vi "Text control 2 v6.4.vi"() -> ()   [LabVIEW 2016]
panel:
  in  "Tab Control":enum32{"Main", "Other parameters"}(tab)
  out "Line running":i32
  out "Total lines":i32
  out "Path":path=path "C:/users/rlp38/09Apr2009LTtesting/test2.txt"
  out "I vs Vg":cluster{"Y data in":dbl[], "X data in":dbl[]}[](graph)
  out "Is max":dbl format="%.2e"
  out "Id max":dbl format="%.2e"
  out "Ig max":dbl format="%.2e"
  out "Imax vs time":cluster{"Y data in":dbl[], "X data in":dbl[]}[](graph)
  out "Imin vs time":cluster{"Y data in":dbl[], "X data in":dbl[]}[](graph)
  out "I vs Vd":cluster{"Y data in":dbl[], "X data in":dbl[]}[](graph)
  in  "Script":string="#pulsedstressV d 0.03 20 0 0.5 0.0827 5\n#\n#itime m\n#gaterangemode a\n#drainrangemode a\n#pulsed on 0.05 0 0.02\n#transfer d -10 40 1 5 40 35\n#transfer d -10 40 1 5 40 35\n#transfer d -10 40 1 5 40 35\n#output d 0 40 20 0 40 1\n#\n#\n#sample 1 0.008 221 6 0.003\n#samplei 400e-6 200 6 0.002 0.1\n#vsu2pulse -10 4\n#\n#stressV 0.016 0.03 2e-4 0.1e-3 11\n#stressI 220e-7 0.08 15\n#transfer s -1 1 0.5 -0.005 0.005 0.005\n#output s 0 0 0 -0.008 0.008 0.002"
  out "Command running:":string
  out "Serial port data":string
  out "Elapsed Time":dbl caption="Elapsed Time (s)"
  in  "Time Units":u16(ring)=1 items=["Seconds", "Minutes", "Hours"]
  in  "Time Offset":dbl caption="Set Start Time (s)"
  in  "Reset":bool
  in  "Auto Reset":bool
  in  "integration time":u32(slide) max=2 step=1 scale=0.0..2.0
  out "Is on":dbl format="%.2e"
  out "Id on":dbl format="%.2e"
  out "Ig on":dbl format="%.2e"
  out "Ion vs time":cluster{"Y data in":dbl[], "X data in":dbl[]}[](graph)
  out "Ioff vs time":cluster{"Y data in":dbl[], "X data in":dbl[]}[](graph)
  out "Ig min":dbl format="%.2e"
  out "Id min":dbl format="%.2e"
  out "Is min":dbl format="%.2e"
  out "Is off":dbl format="%.2e"
  out "Id off":dbl format="%.2e"
  out "Ig off":dbl format="%.2e"
  in  "Integration time (long)":dbl=0.32 min=0.04 max=2.0 step=0.02 format="%.2f"
  in  "Integration time (short)":dbl=0.0019 min=8e-05 max=0.0019 step=8e-05 format="%^.0e"
  in  "Drain: Compliance":dbl=0.001 format="%.8f"
  in  "Gate: Compliance":dbl=0.001 format="%.8f"
  in  "Interrupt scan":bool
  in  "Interrupt program":bool
  in  "Plot output curve extrema vs time":bool
  in  "Plot transfer curve extrema vs time":bool
  in  "Gate Range\nmode":u16(ring) items=["Auto", "Limited", "Fixed"]
  in  "Gate Range":u8(slide)=6 max=11 scale=0.0..11.0
  in  "Source/Drain\nRange mode":u16(ring) items=["Auto", "Limited", "Fixed"]
  in  "Source/Drain Range":u8(slide)=6 max=11 scale=0.0..11.0
  in  "Panel Controls":T1={"Emergency Stop"=refnum, "TransGraph Max"=1e-05, "Text/Graph (text=false)"=TRUE} {"TransGraph Max" format="%.2e"}
  in  "Panel Controls 2":T2={"Emergency Stop"=refnum, "TransGraph Max"=1e-05, "Text/Graph (text=false)"=TRUE, "TransGraph Min"=1e-11} {"TransGraph Min" format="%.2e"; "TransGraph Max" format="%.2e"}
  out "error out":errorcluster
  in  "Delay before read (ms)":u32=1000
  in  "byte count":u32=64
  in  "Serial End Mode for Reads":u16(ring)=2 items=["None", "LastBit", "TermChar"]
  in  "Timeout (ms)":u32=10000
  in  "Enable Termination\nChar (T)":bool=TRUE
  in  "Termination char\n(0xA = '\\n' = LF)\n(0xD = '\\r' = CR)":u8=13 format="%.0x"
  in  "flow control":u16(ring) items=["None"=0, "XON/XOFF"=1, "RTS/CTS"=2, "DTR/DSR"=4]
  in  "stop bits":u16(ring)=10 items=["1.0"=10, "1.5"=15, "2.0"=20]
  in  "parity":u16(ring) items=["None", "Odd", "Even", "Mark", "Space"]
  in  "data bits":u16=8 min=5 max=8 step=1
  in  "VISA resource name":refnum<visa-resource-name>="COM6"
  in  "baud rate":u32=9600
  out "Timings Indicator":T3
  in  "Timings (overwritten by the Front Panel)":T4={"integration time"=0, "Short/Long integration time"=0.00064, "hold time (sec)"=0.0, "delay time (sec)"=0.0, "Step Time (0 disables)"=0.0, "sweep method"=0, "Pulse period"=0.005, "Base voltage"=0.0, "Pulse width"=0.0005} {"Pulse width" min=0.0005 max=0.1 step=0.0001 format="%.4f"; "Base voltage" format="%^.4e"; "Pulse period" min=0.005 max=1.0 step=0.0001 format="%.4f"; "sweep method" items=["Continuous", "Pulsed"]; "Step Time (0 disables)" format="%.2f"; "delay time (sec)" format="%.4f"; "hold time (sec)" format="%.4f"; "Short/Long integration time" format="%^.0e"; "integration time" scale=0.0..2.0}
  in  "SMU4":cluster{"on/off":bool, "Voltage":dbl} {"Voltage" min=-100.0 max=100.0 format="%.2f"}
  in  "Full Reset":bool
  in  "Standby":T5
  in  "Gate":T6={"Gate Start"=0.0, "Gate Stop"=2.0, "Gate Step (linear only)"=1.0, "Gate Compliance"=0.0001, "Gate PComp"=0.0, "Range mode"=0, "Range"=6} {"Range" max=11 scale=0.0..11.0; "Range mode" items=["Auto", "Limited", "Fixed"]; "Gate PComp" format="%^.2e"; "Gate Compliance" format="%^.2e"; "Gate Step (linear only)" format="%^.4e"; "Gate Stop" format="%^.4e"; "Gate Start" format="%^.4e"}
  in  "Drain 2":T7={"Drain Start"=0.0, "Drain Stop"=2.0, "Drain Compliance"=0.0001, "Drain Step"=1.0, "Drain PComp"=0.0, "Range mode"=0, "Range"=6} {"Range" max=11 scale=0.0..11.0; "Range mode" items=["Auto", "Limited", "Fixed"]; "Drain PComp" format="%^.2e"; "Drain Step" format="%^.4e"; "Drain Compliance" format="%^.2e"; "Drain Stop" format="%^.4e"; "Drain Start" format="%^.4e"}
  # "Time"
  # "Syntax:\nitime [s|m|l] time(sec): [s|m|l] determines the integration time setting (small|medium|long) and time sets the value.\nNOTE: The value of the integration time has to be within the range allowed by its category (s|m|l), otherwise, the closest value will be used. (e.g. if the category is set to short but the time value is very long, the actual value used will be the maximum short integration time.\nIntegration times:\n    Short: Default: 640 us. Range: 8E-5 - 1.92E-3 seconds.\n    Medium: Fixed at 1 NPL cycle (0.02 seconds).\n    Long: Default: 16 NPL cycles (0.32 seconds). Range: 2-100 NPL cycles (0.04 seconds - 2 seconds).\ngaterangemode [a|l|f]\ndrainrangemode [a|l|f]\npulsed [on|off] PulsePeriod(sec) PulseBaseVoltage PulseONWidth(sec)\nstandby [on l off]\nwait NumMilliseconds\nwait-min NumMinutes\n# texthere = comment\ntransfer [s|d] VgStart VgStop VgStep VdStart VdStop VdStep\noutput [s|d] VgStart VgStop VgStep VdStart VdStop VdStep\nsample Vg Vd NumSamples Time(s) SampleInterval(s)\nsamplei Idg NumSamples Time(s) SampleInterval(s) VDGcompliance\n100 samples is approximately 13 seconds with medium integration\n# if in doubt use SampleInterval(s) = 0.004\nstressV VG VD IGcompliance IDcompliance Duration(sec)\nstressI IDG VDGcompliance Duration(sec)\nvsu2pulse Bias Duration(s)\npulsedstressV [s|d] VEstop VgON VgOFF Period(s) PulseONwidth(s) Vd\nsample-fpp Vg Vd NumSamples Time\nresample-fpp Vg Vd\ntransfer-fpp [s|d] VgStart VgStop VgStep VdStart VdStop VdStep\noutput-fpp [s|d] VgStart VgStop VgStep VdStart VdStop VdStep\nserial SerialPortCommand"
  # "1\n2\n3\n4\n5\n6\n7\n8\n9\n10\n11\n12\n13\n14\n15\n16\n17\n18\n19\n20"
  # "Serial port settings"
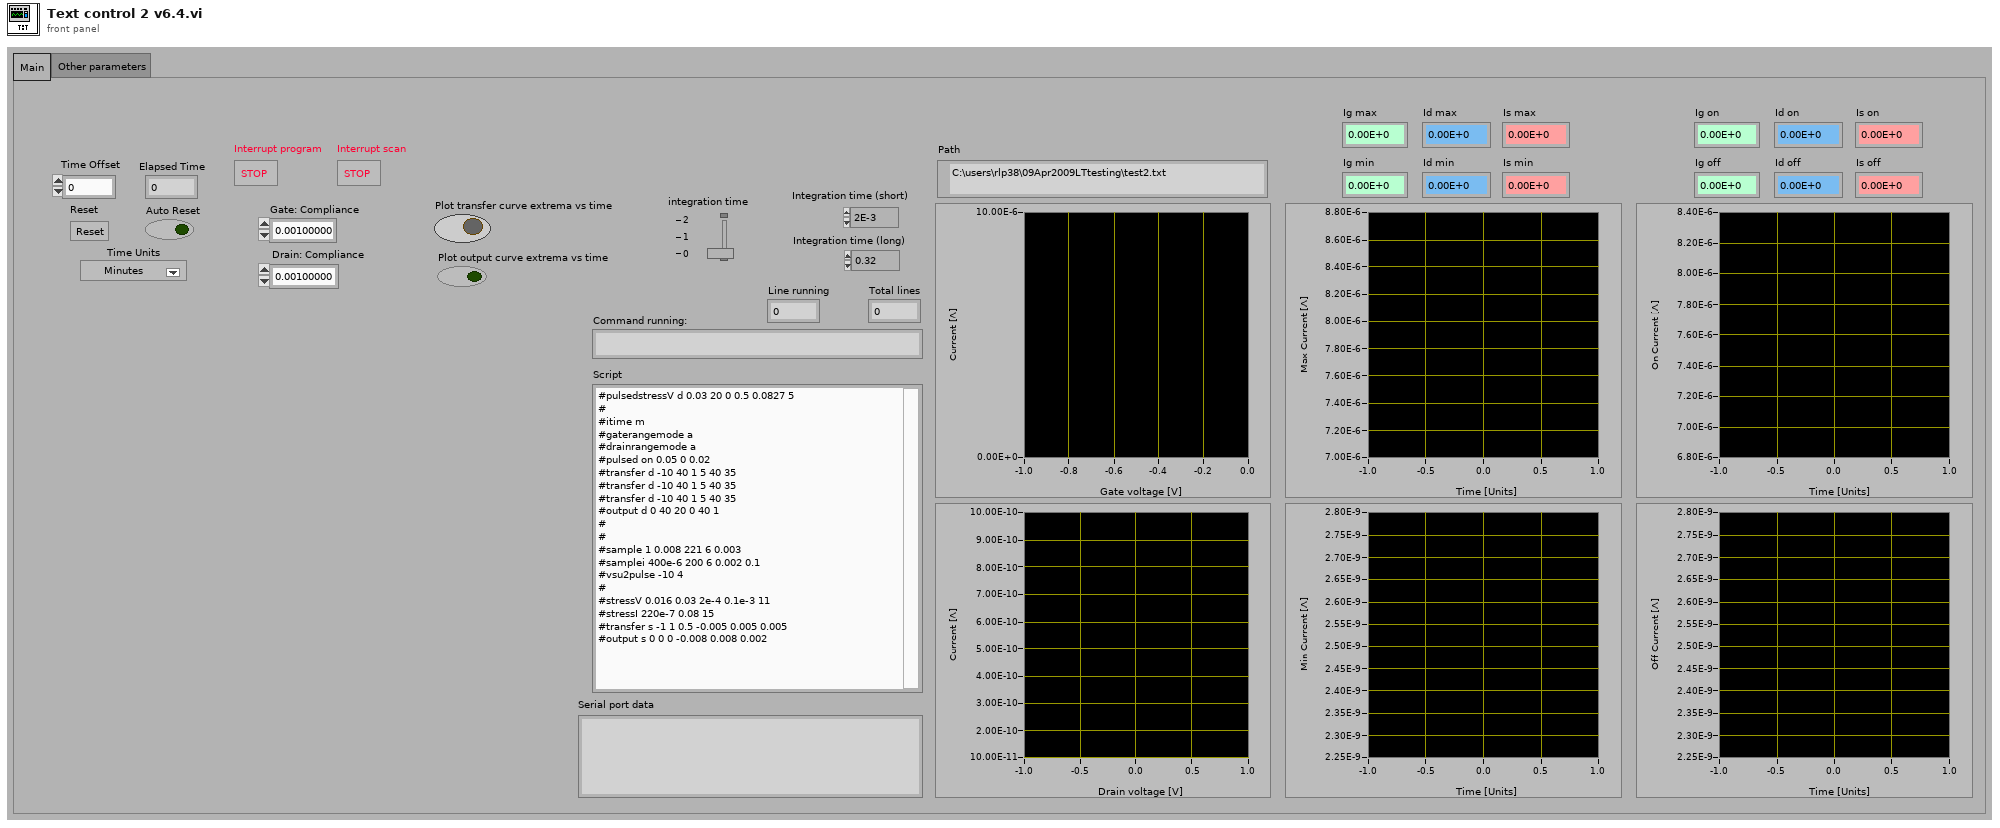
[diagram p1: front panel]
types:
  T1 = cluster{"Emergency Stop":refnum<vi>, "TransGraph Max":dbl, "Text/Graph (text=false)":bool}
  T2 = cluster{"Emergency Stop":refnum<vi>, "TransGraph Max":dbl, "Text/Graph (text=false)":bool, "TransGraph Min":dbl}
  T3 = cluster{"integration time (0:s, 1:m, 2:l)":u32, "Short/Long integration time":dbl, "hold time (sec)":dbl, "delay time (sec)":dbl, "Step Time (0 disables)":dbl, "sweep method":u16, "Pulse period":dbl, "Base voltage":dbl, "Pulse width":dbl}
  T4 = cluster{"integration time":u32, "Short/Long integration time":dbl, "hold time (sec)":dbl, "delay time (sec)":dbl, "Step Time (0 disables)":dbl, "sweep method":u16, "Pulse period":dbl, "Base voltage":dbl, "Pulse width":dbl}
  T5 = cluster{"Gate Standby":bool, "Drain Standby":bool}
  T6 = cluster{"Gate Start":dbl, "Gate Stop":dbl, "Gate Step (linear only)":dbl, "Gate Compliance":dbl, "Gate PComp":dbl, "Range mode":u16, "Range":u8}
  T7 = cluster{"Drain Start":dbl, "Drain Stop":dbl, "Drain Compliance":dbl, "Drain Step":dbl, "Drain PComp":dbl, "Range mode":u16, "Range":u8}
  T8 = enum16{"open", "replace", "create", "open or create", "replace or create", "replace or create with confirmation"}
  T9 = cluster{"V2 Start":dbl, "V2 Step":dbl, "Number of points":i32}
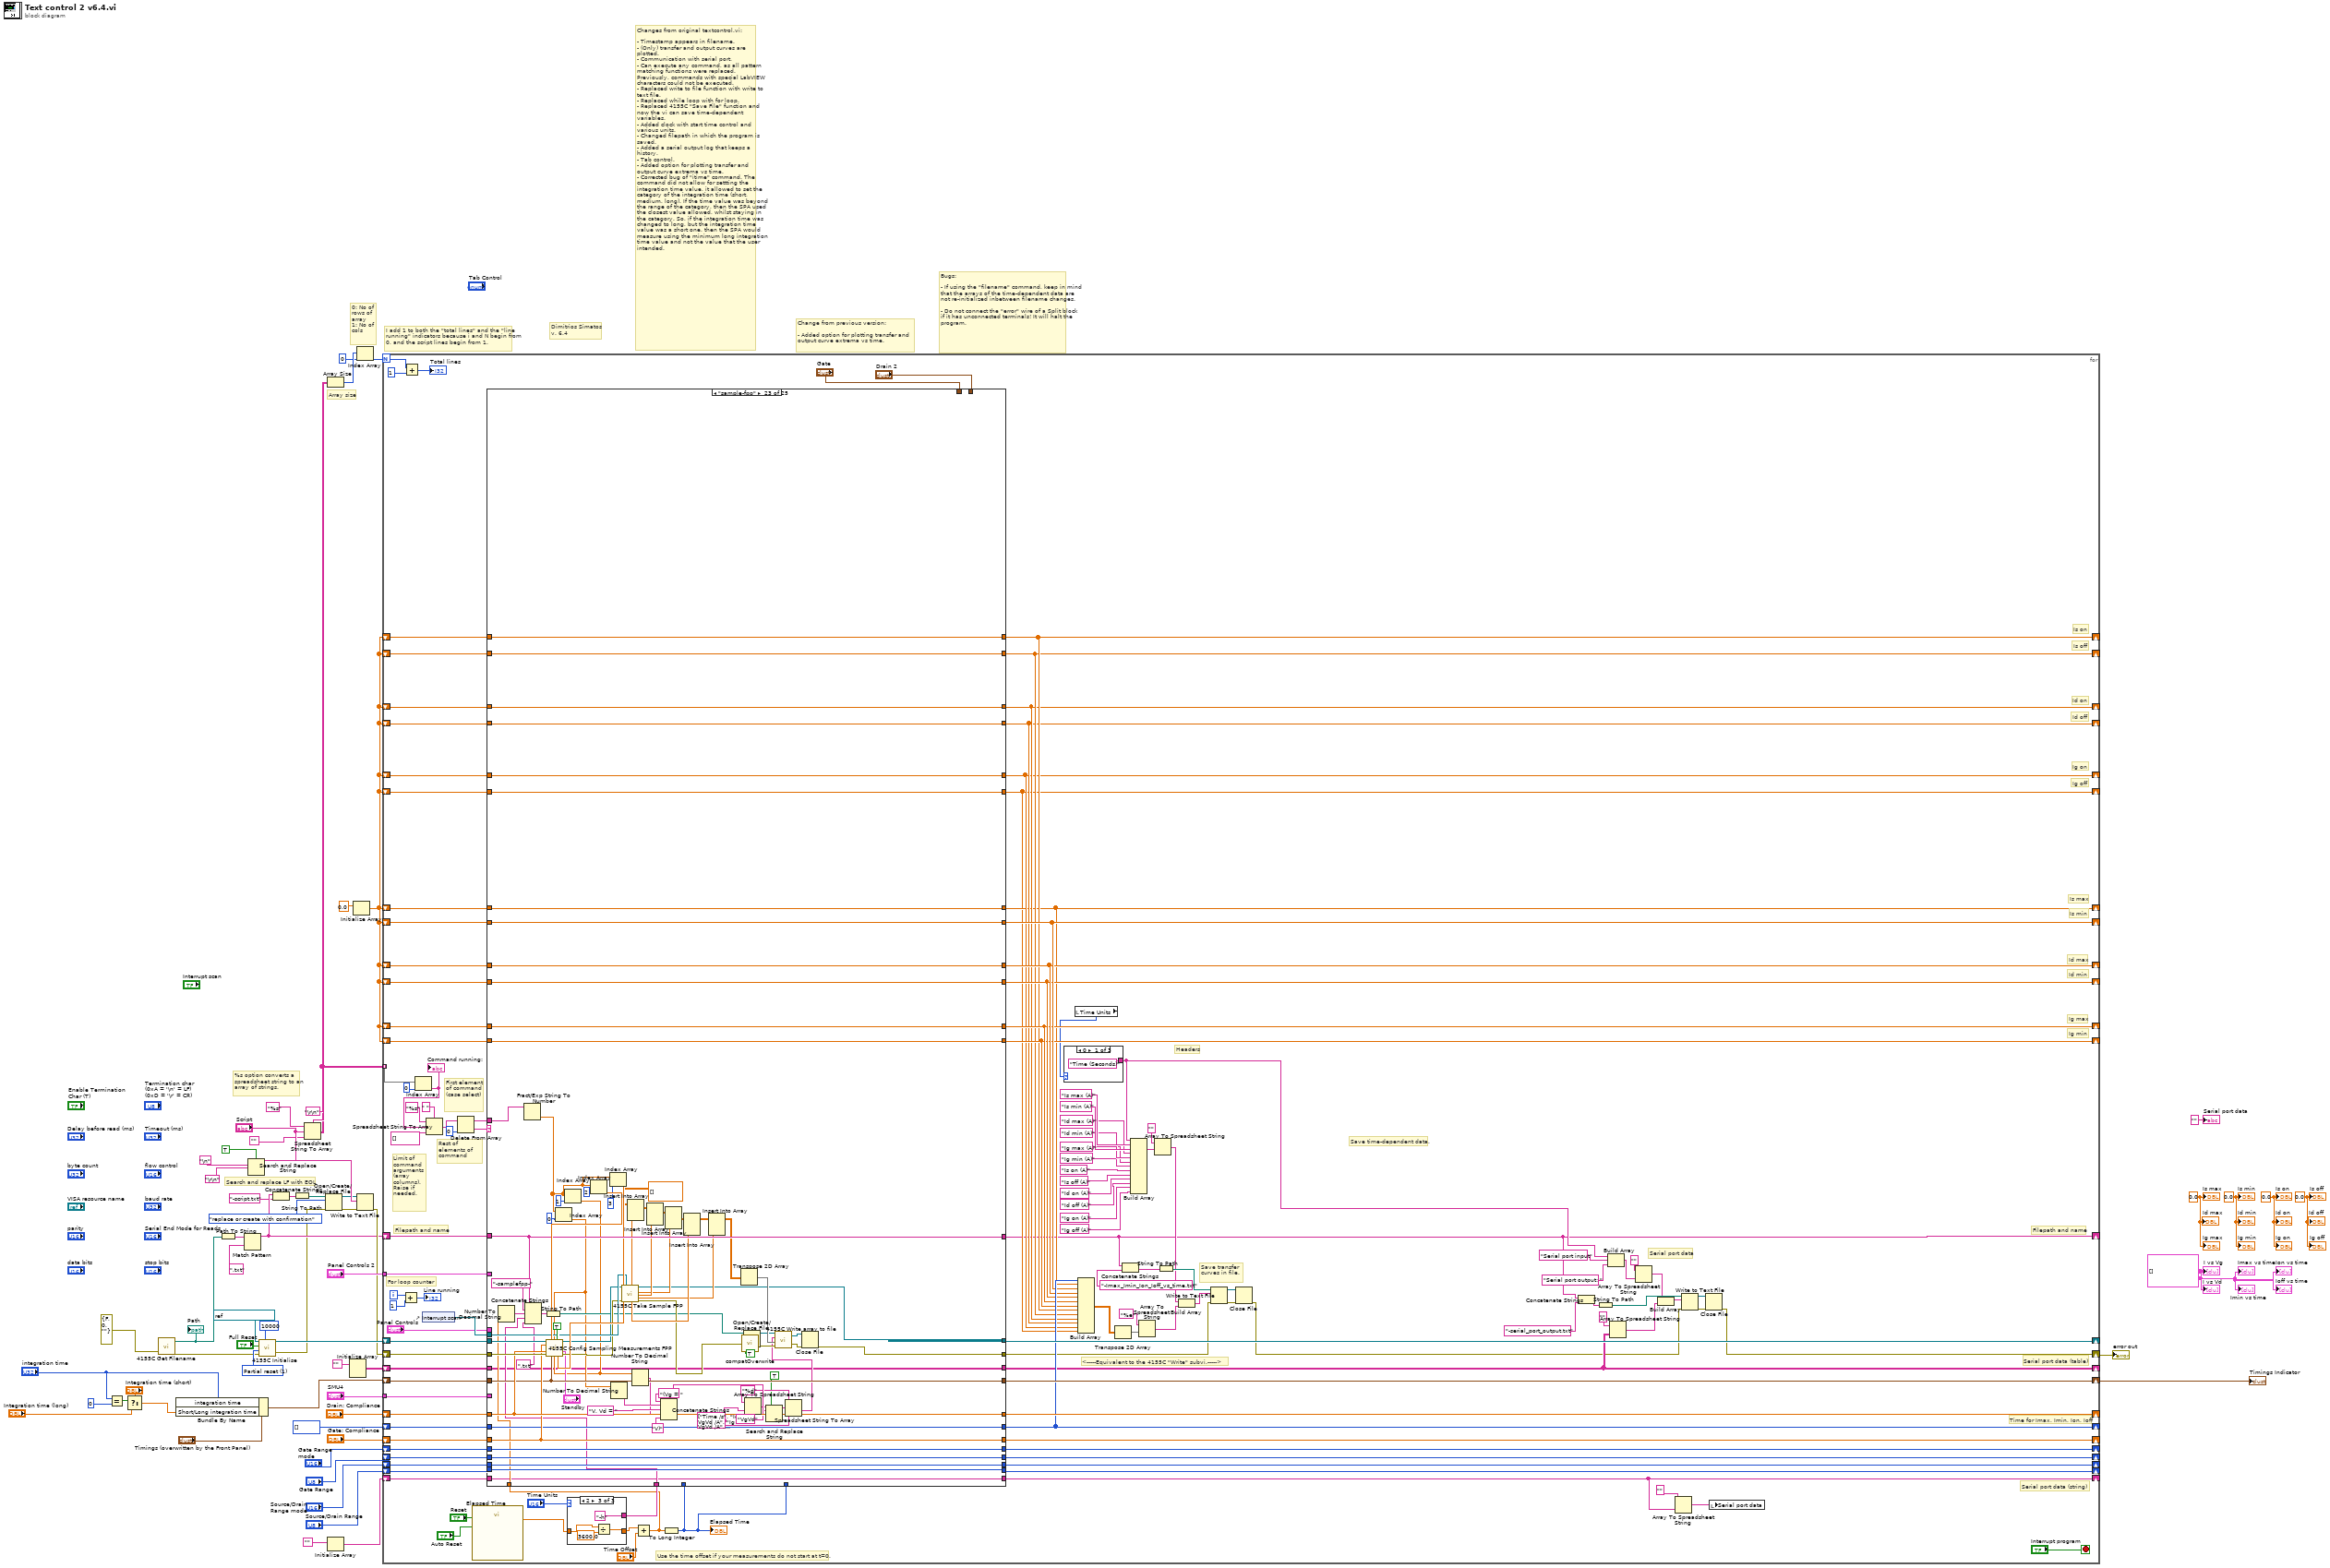
[diagram p0: block diagram]
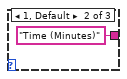
[diagram p2: hidden frame]
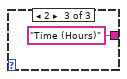
[diagram p3: hidden frame]
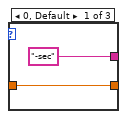
[diagram p4: hidden frame]
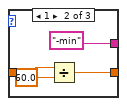
[diagram p5: hidden frame]
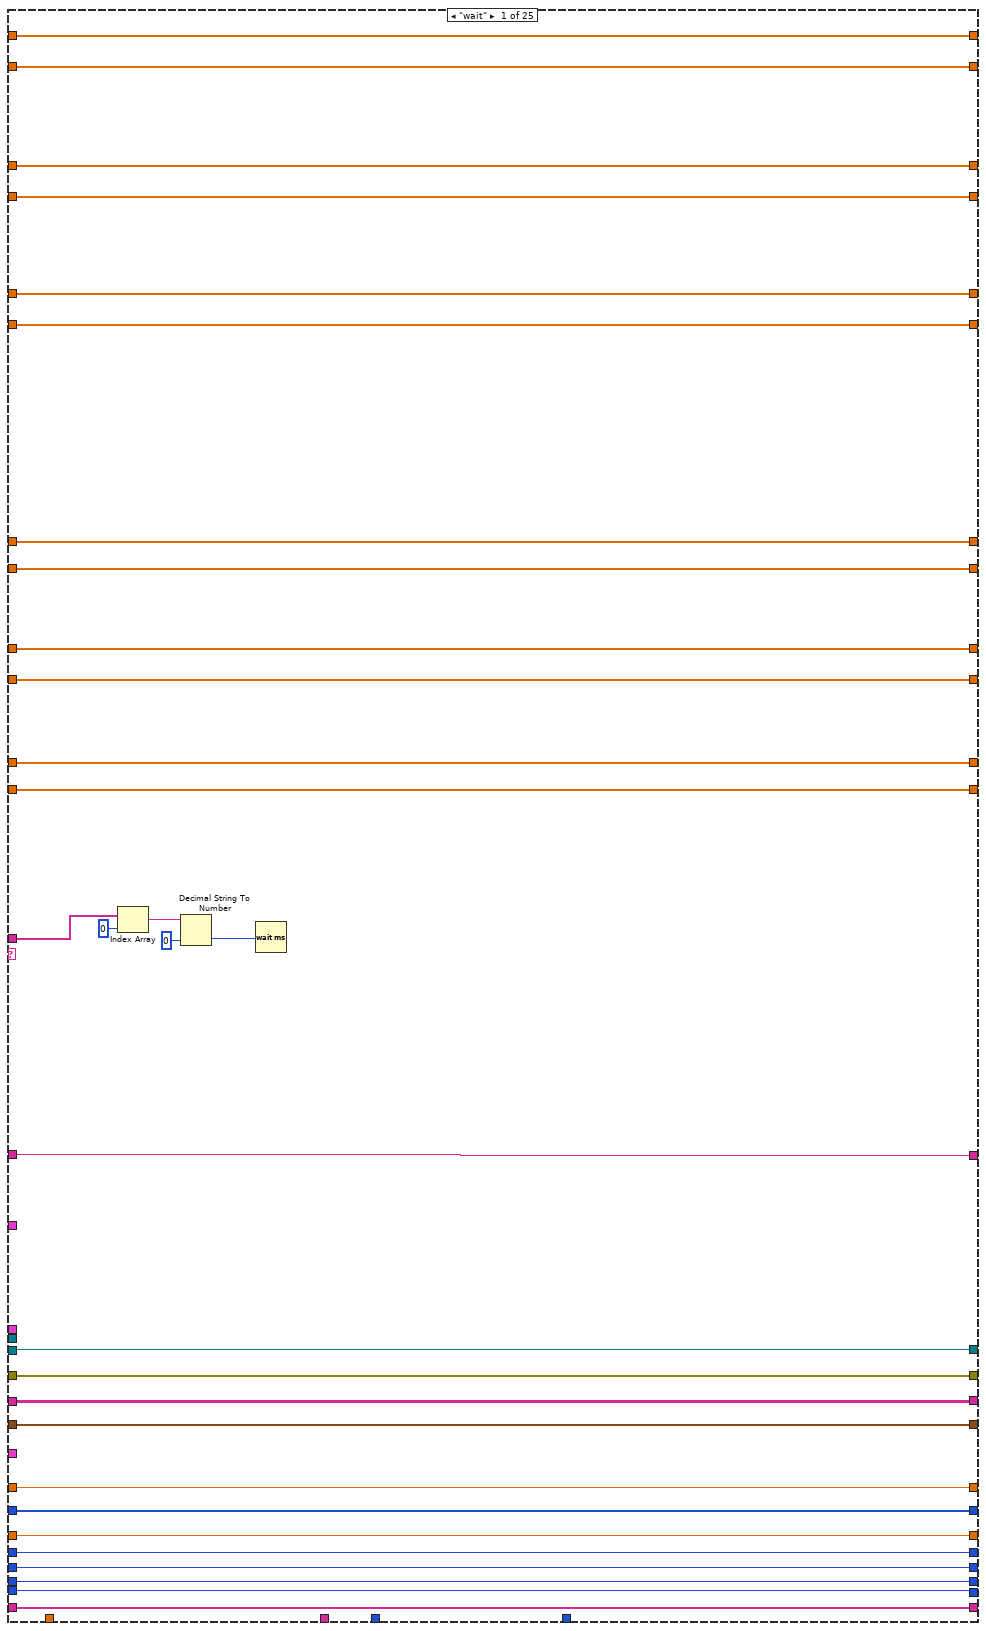
[diagram p6: hidden frame]
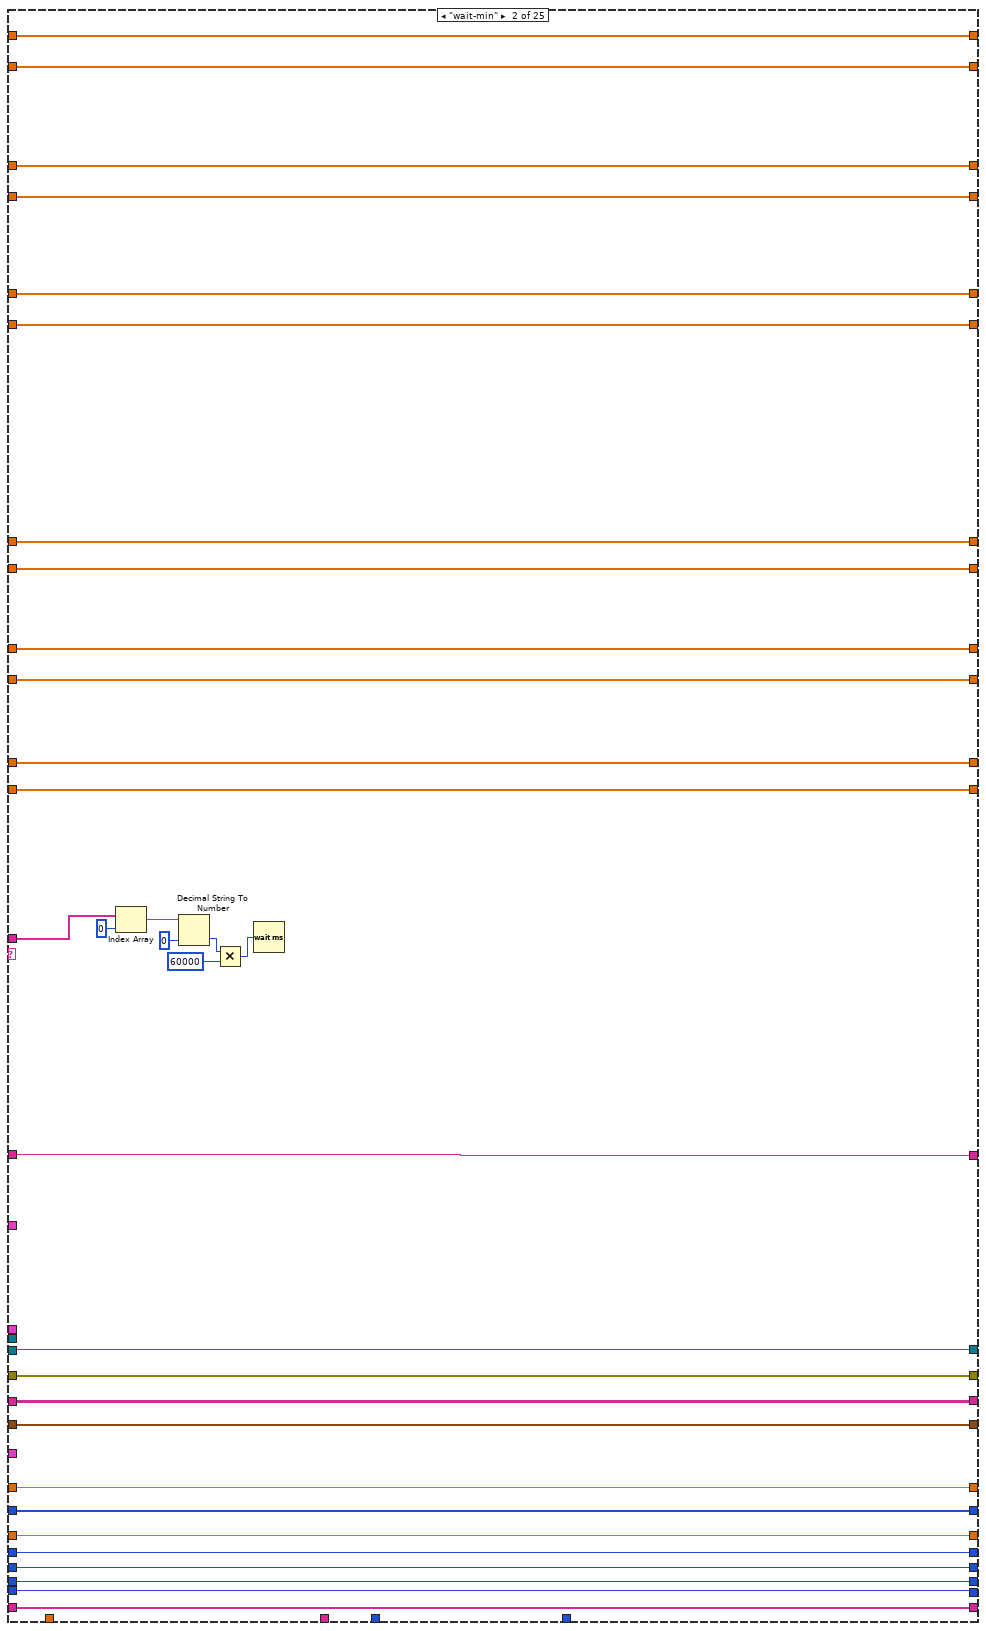
[diagram p7: hidden frame]
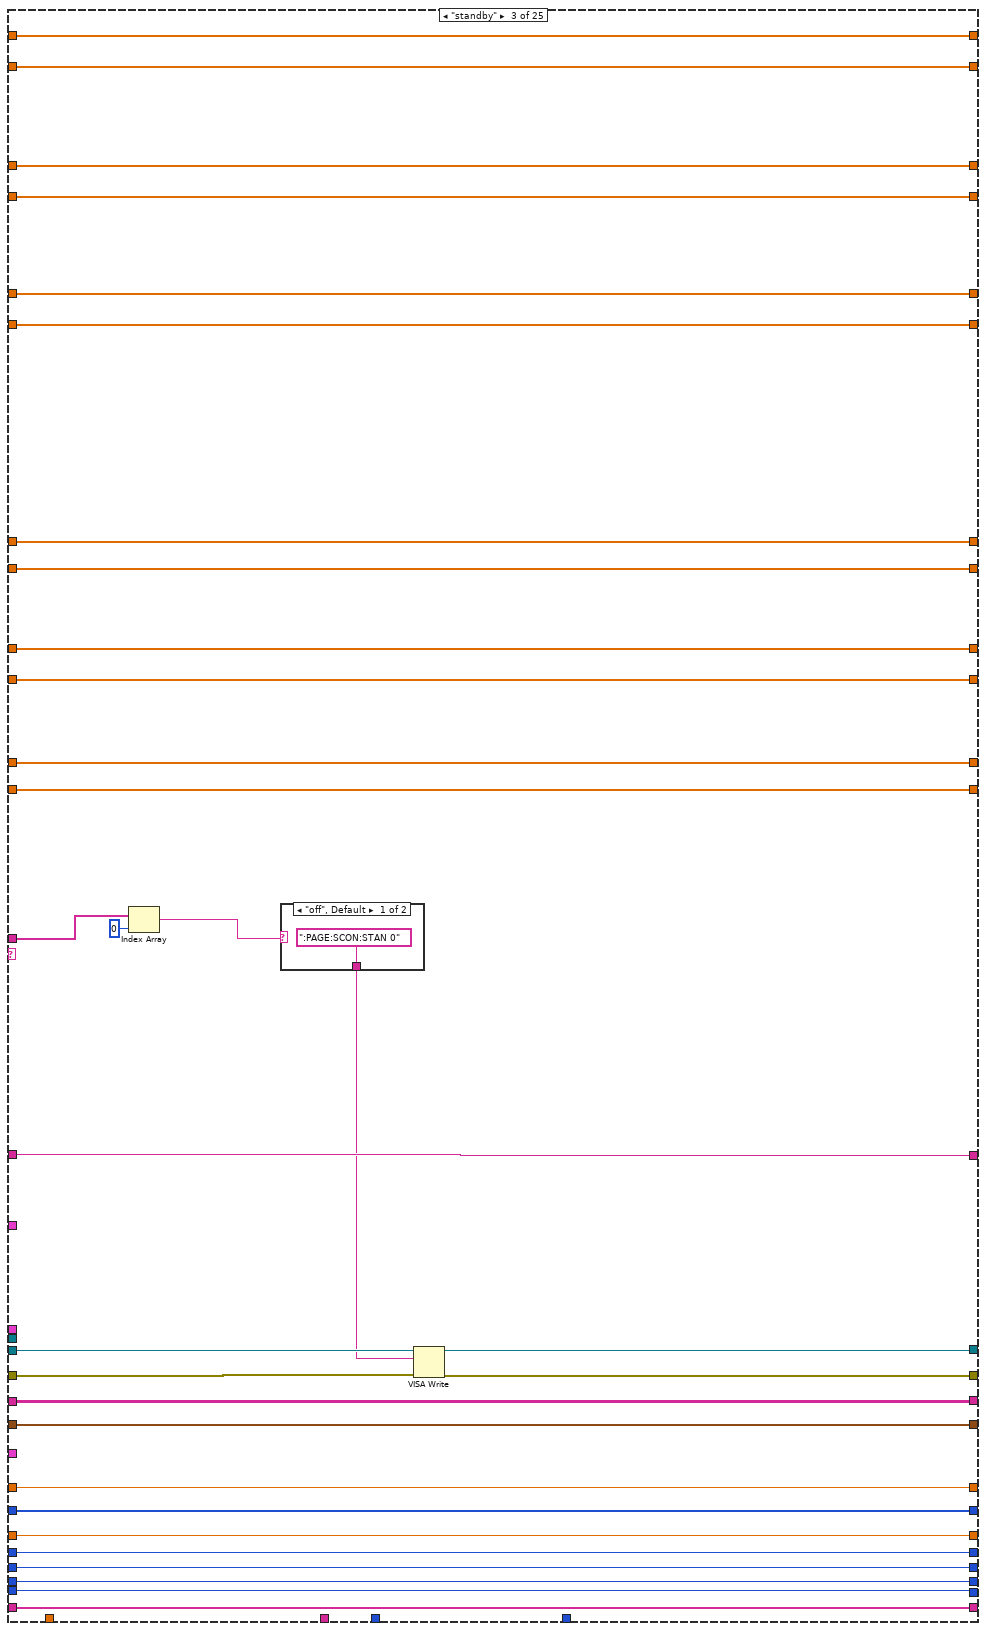
[diagram p8: hidden frame]
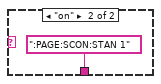
[diagram p9: hidden frame]
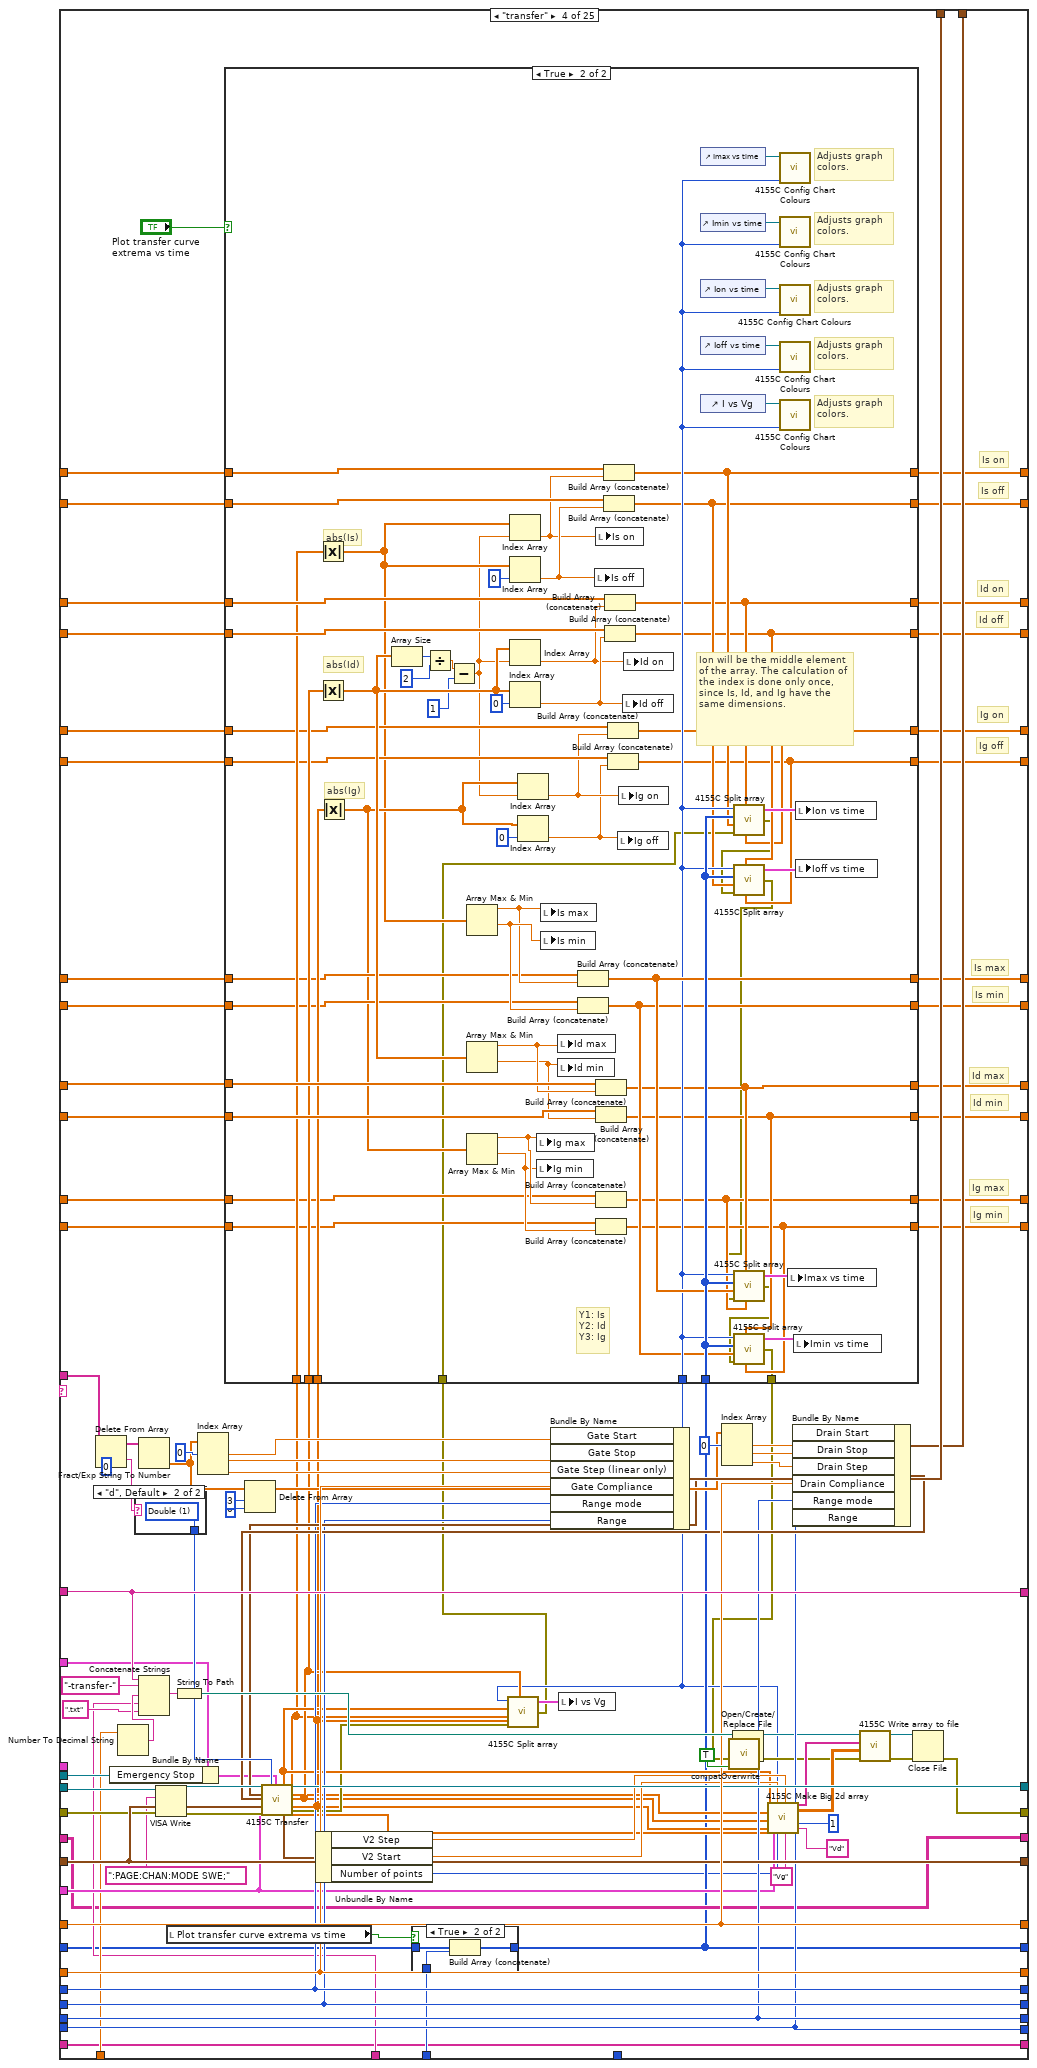
[diagram p10: hidden frame]
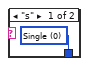
[diagram p13: hidden frame]
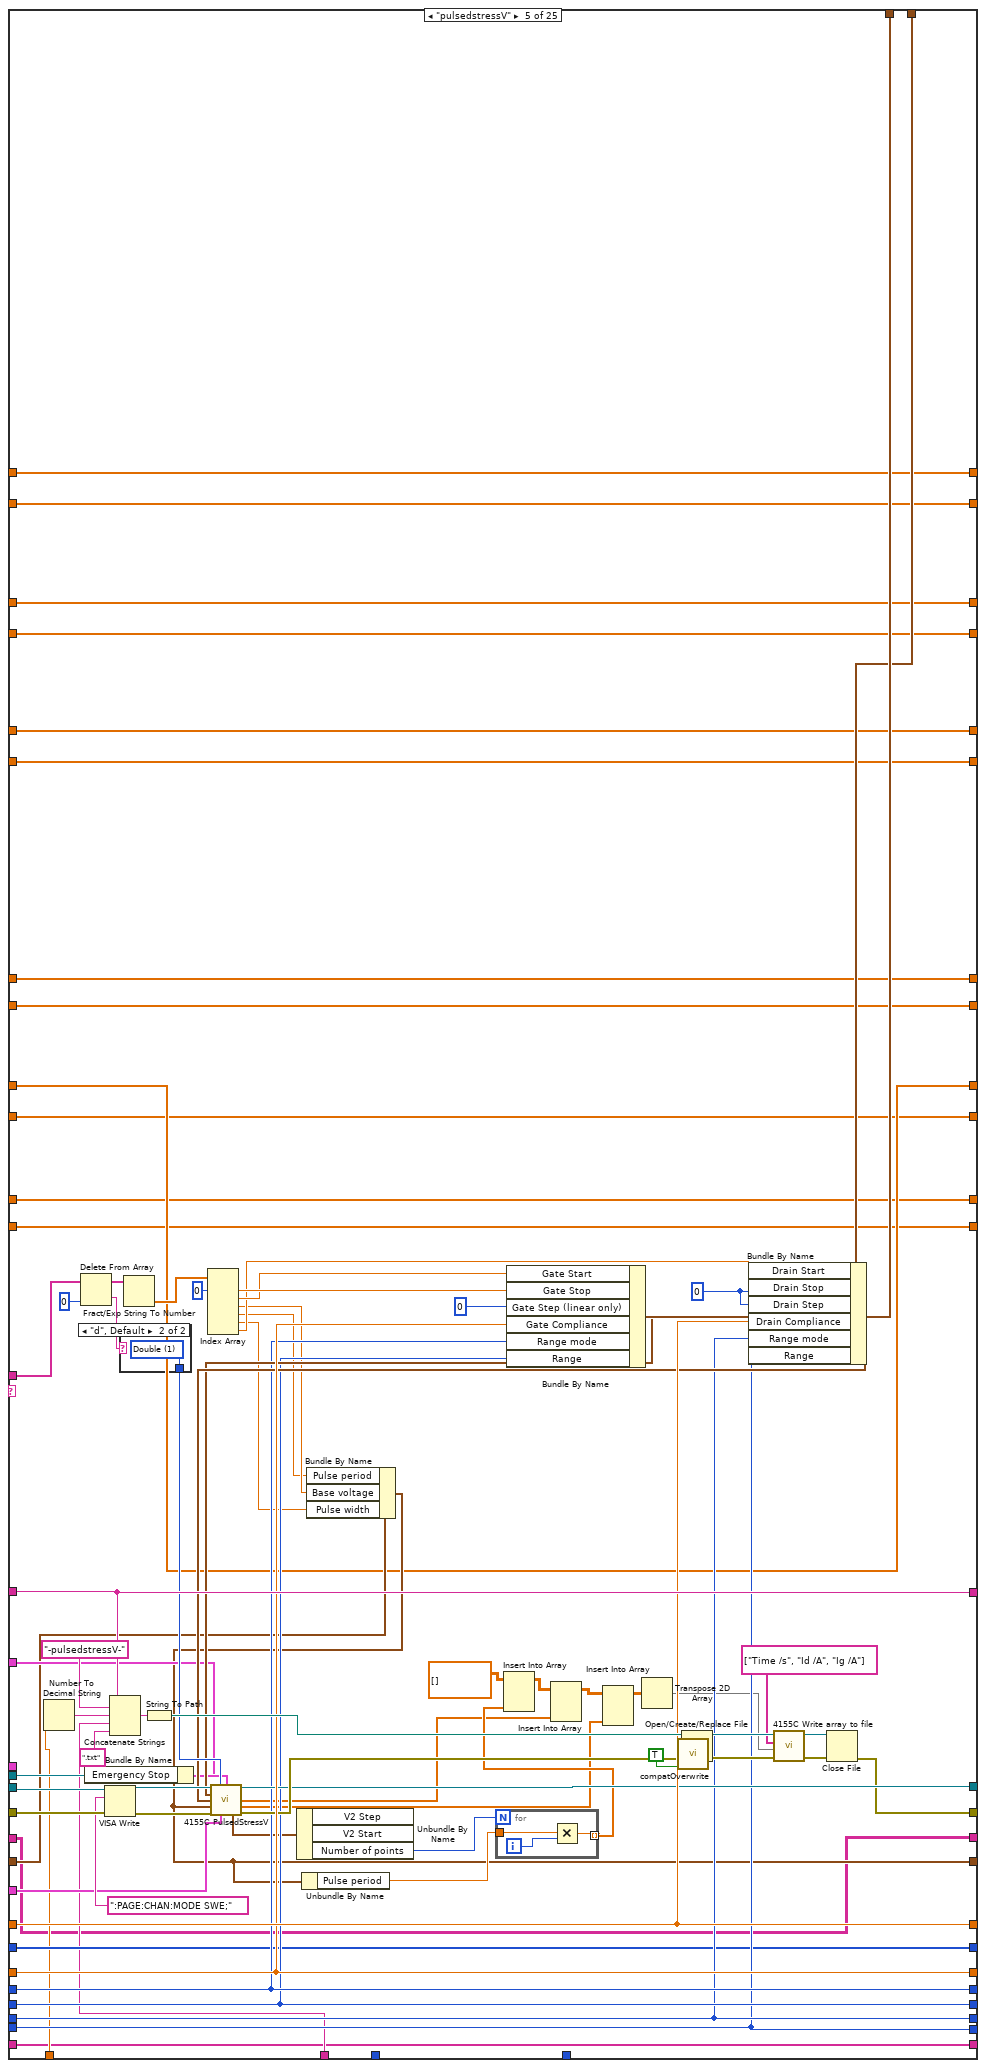
[diagram p14: hidden frame]
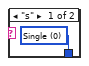
[diagram p15: hidden frame]
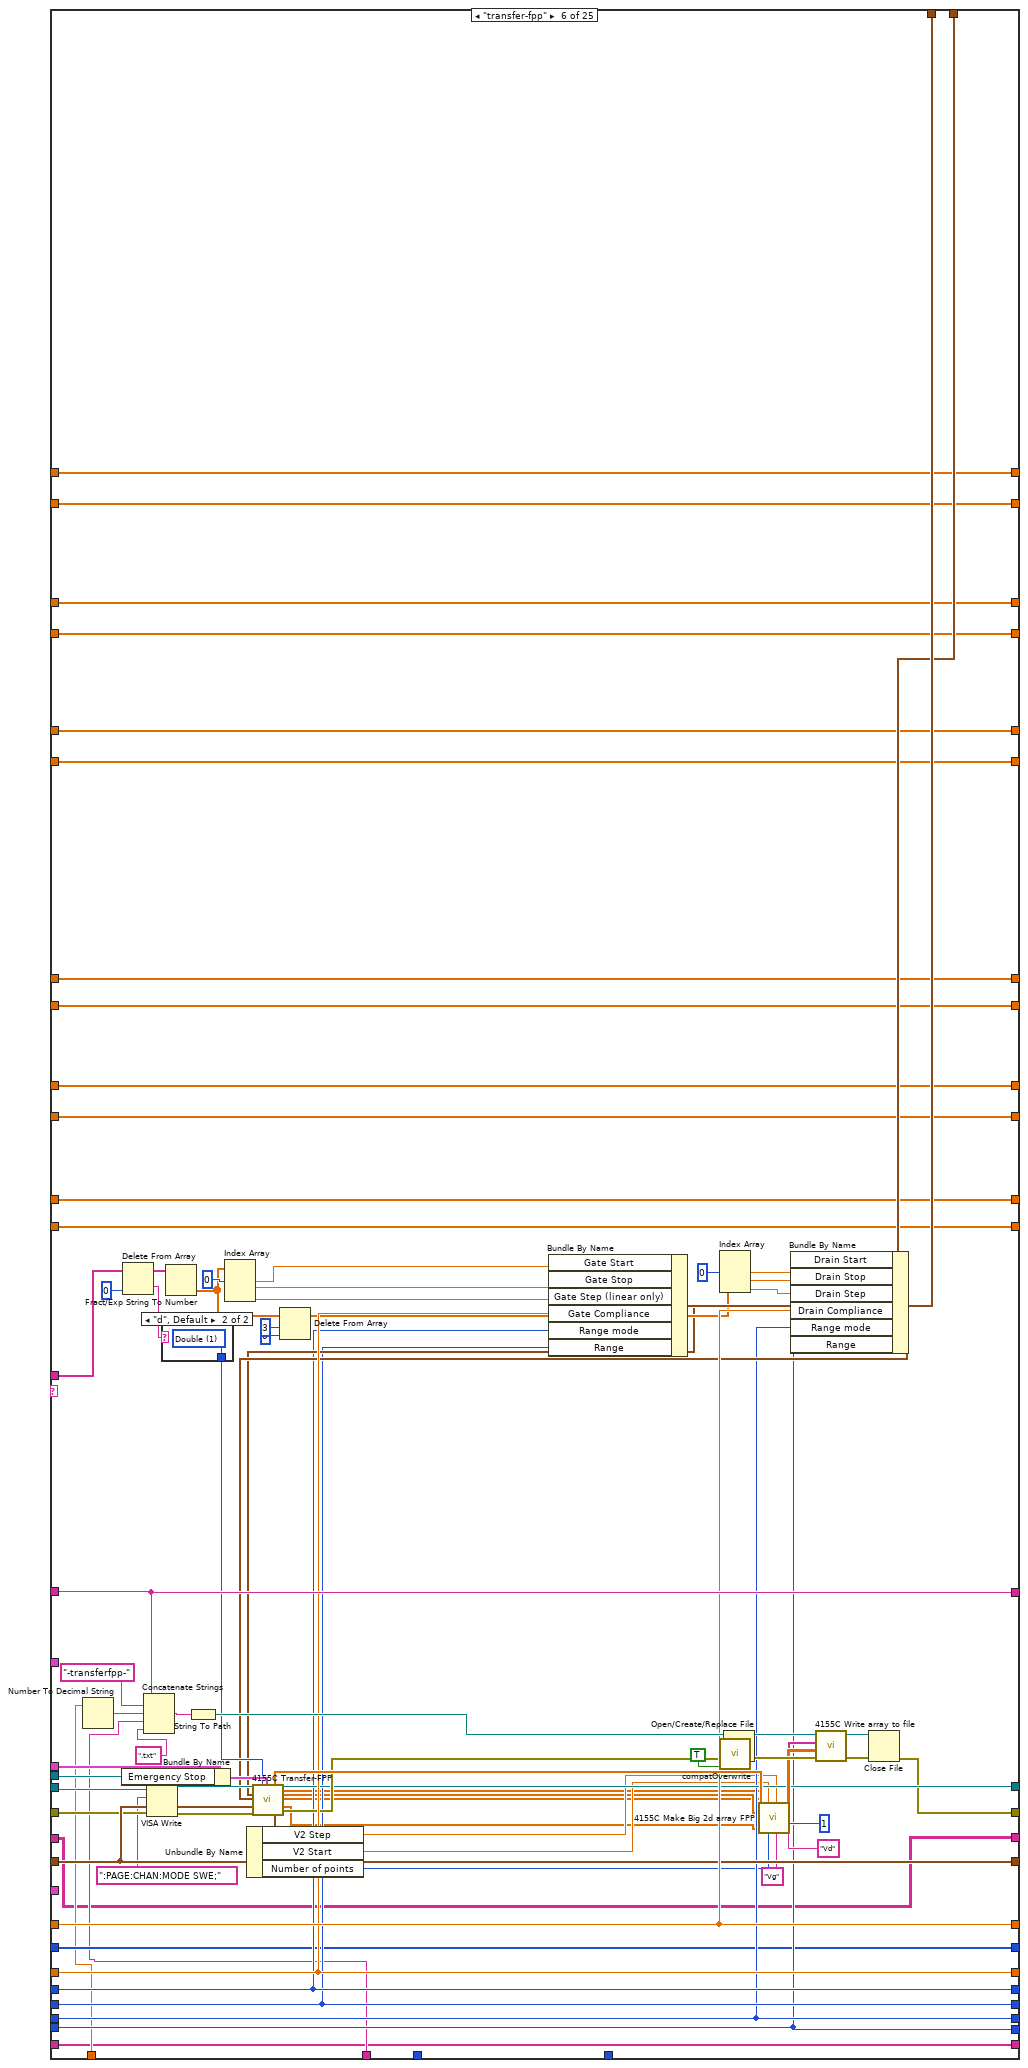
[diagram p16: hidden frame]
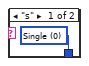
[diagram p17: hidden frame]
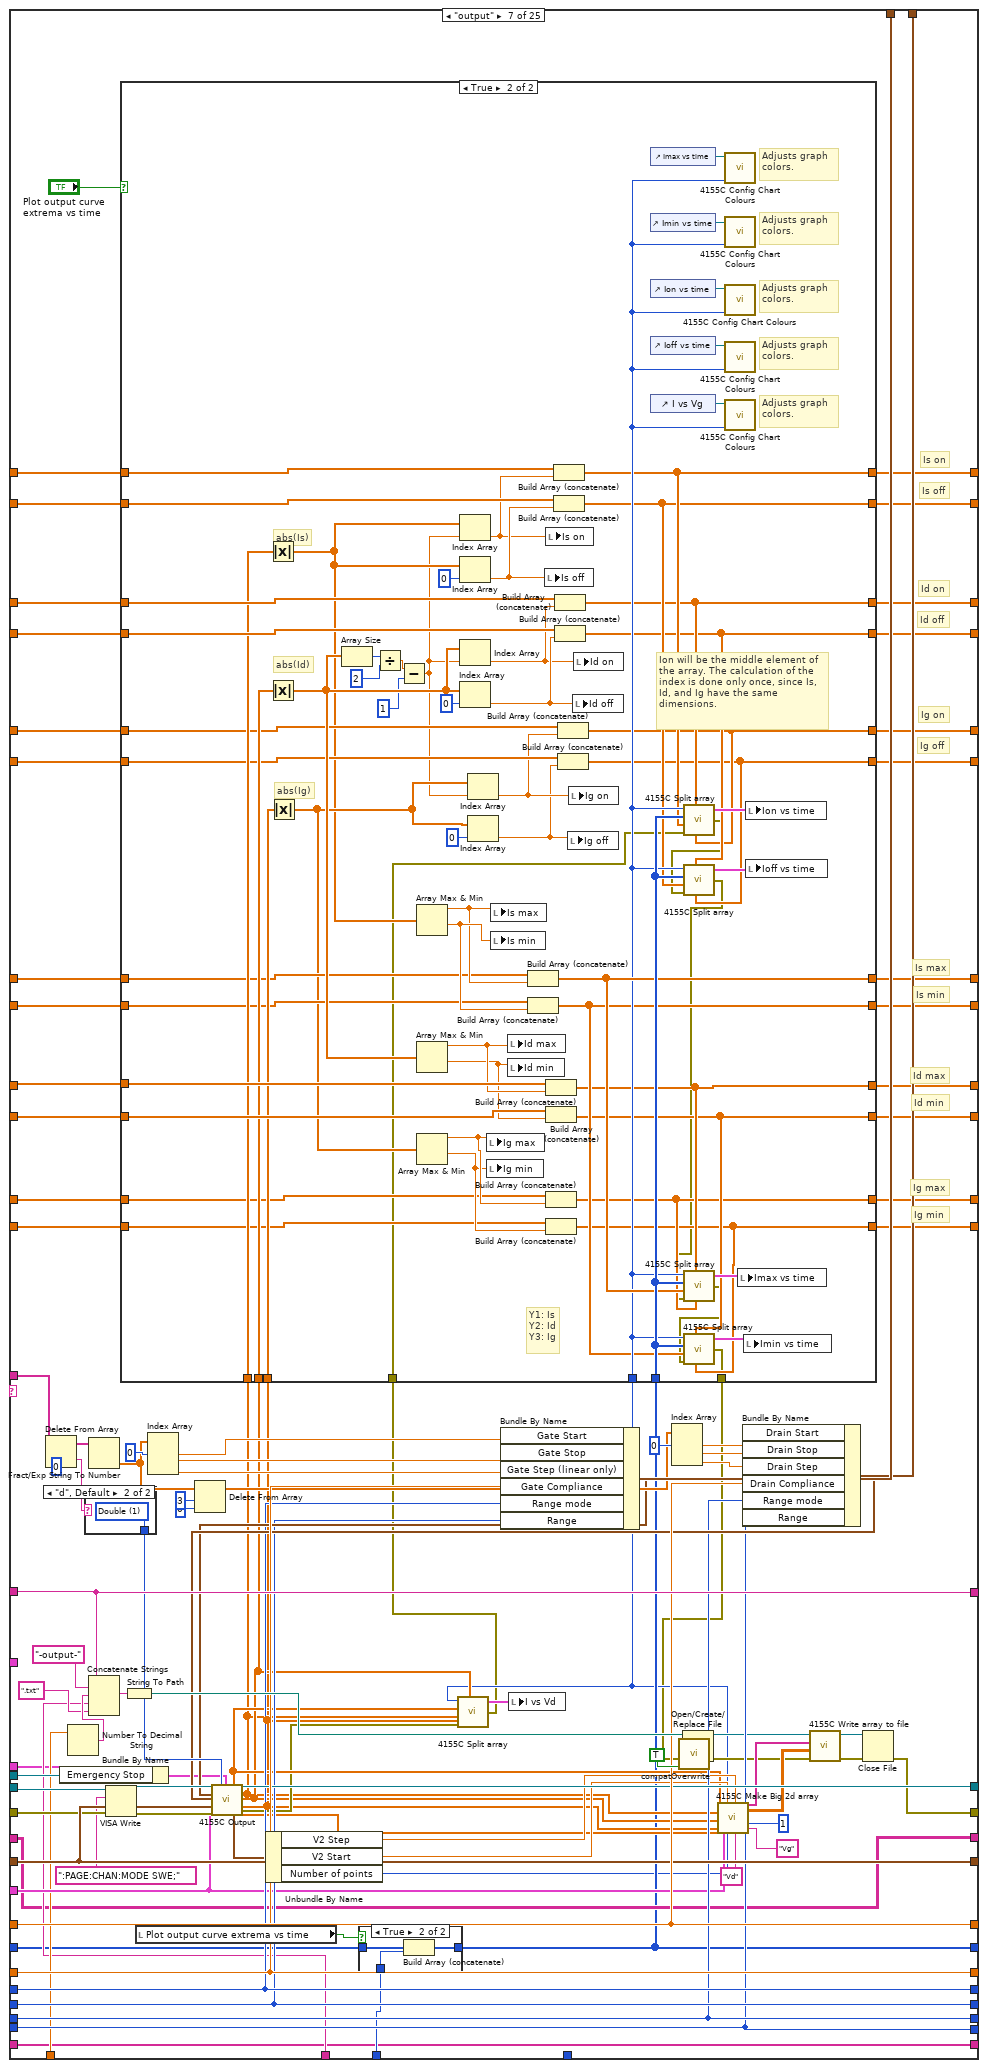
[diagram p18: hidden frame]
diagram:
  w7 = cluster{"Y data in":dbl[], "X data in":dbl[]}[] [] ("I vs Vg")
  w8 = 0.0 ("Is off")
  w9 = 0.0 ("Is on")
  w10 = 0.0 ("Is min")
  w11 = 0.0 ("Is max")
  w57 = u16 1 items=["Reset All", "Partial reset"] ("Type of reset")
  # "Change from previous version:\n\n- Added option for plotting transfer and output curve extrema vs time."
  # "I add 1 to both the \"total lines\" and the \"line running\" indicators because i and N begin from 0, and the script lines begin from 1."
  # "Bugs:\n\n- If using the \"filename\" command, keep in mind that the arrays of the time-dependent data are not re-initialized inbetween filename changes. \n\n- Do not connect the \"error\" wire of a Split block if it has unconnected terminals! It will halt the program."
  # "Array size"
  # "%s option converts a spreadsheet string to an array of strings."
  # "0: No of rows of array\n1: No of cols"
  # "Dimitrios Simatos\nv. 6.4"
  # "Changes from original textcontrol.vi:\n\n- Timestamp appears in filename.\n- (Only) transfer and output curves are plotted.\n- Communication with serial port.\n- Can execute any command, as all pattern matching functions were replaced. Previously, commands with special LabVIEW characters could not be executed.\n- Replaced write to file function with write to text file.\n- Replaced while loop with for loop.\n- Replaced 4155C \"Save File\" function and now the vi can save time-dependent variables.\n- Added clock with start time control and various units.\n- Changed filepath in which the program is saved.\n- Added a serial output log that keeps a history.\n- Tab control.\n- Added option for plotting transfer and output curve extrema vs time.\n- Corrected bug of \"itime\" command. The command did not allow for settting the integration time value, it allowed to set the category of the integration time (short, medium, long). If the time value was beyond the range of the category, then the SPA used the closest value allowed, whilst staying in the category. So, if the integration time was changed to long, but the integration time value was a short one, then the SPA would measure using the minimum long integration time value and not the value that the user intended."
  # "Search and replace LF with EOL"
  n1 = Equal?(x="integration time", y=u32 0) -> (x = y?=w58:bool)
  n2 = Select(t="Integration time (short)", s=w58, f="Integration time (long)") -> (s? t:f=w16:dbl)
  n3 = call "4155C Get Filename.vi"("error in (no error)"=errorcluster {"status"=FALSE, "code"=0, "source"=""}) -> ("error out"=w52:errorcluster, "path"=w27:path)  [unwired: 2 in, 1 out]
  "Path" <- w27
  n4 = Bundle By Name(cluster="Timings (overwritten by the Front Panel)", "integration time"="integration time", "Short/Long integration time"=w16) -> (w50:T4)
  n5 = Path To String(path=w27) -> (string=w28:string)
  n6 = Match Pattern(string=w28, regular expression=".txt") -> (before substring=w14:string)  [unwired: 1 in, 3 out]
  n7 = Search and Replace String(replace all?=TRUE ("replace all? (F)"), input string="Script", search string="\n", replace string="\r\n") -> (result string=w40:string)  [unwired: 4 in, 3 out]
  n8 = call "4155C Initialise.vi"("VISA resource name in"=refnum<visa-resource-name> "GPIB0::14::INSTR", "Reset"="Full Reset", "Type of reset"=w57, "error in (no error)"=w52, "VISA Timeout Value"=u32 10000) -> ("VISA Resource Name out"=w51:refnum<visa-resource-name>, "error out"=w5:errorcluster)
  n9 = Concatenate Strings(w14, "-script.txt" ("string")) -> (w15:string)
  n10 = String To Path(string=w15) -> (path=w3:path)
  n11 = Spreadsheet String To Array(delimiter (Tab)="\r\n", format string="%s", spreadsheet string="Script", array type (2D Dbl)="") -> (array=w31:string[][])
  n12 = Open/Create/Replace File(file path (use dialog)=w3, error in=w5, operation (0:open)=T8."replace or create with confirmation") -> (refnum out=w2:refnum<file>, error out=w4:errorcluster)  [unwired: 3 in, 1 out]
  n13 = Array Size(array=w31) -> (size(s)=w35:i32[])
  n14 = Initialize Array("") -> (w20:string[])  [unwired: 1 in]
  n15 = Initialize Array("") -> (w18:string[][])  [unwired: 2 in]
  n16 = Initialize Array(0.0 ("element")) -> (w22:dbl[])  [unwired: 1 in]
  n17 = Index Array(array=w35, index=0) -> (element=w33:i32)
  n18 = Write to Text File(file (use dialog)=w2, text=w40, error in=w4) -> (error out=w24:errorcluster)  [unwired: 1 in, 2 out]
  n19 = for {
    N: w33 -> [w130]
    tunnel: "SMU4" -> [w166]
    shift-left: "Source/Drain Range" -> [w171]
    shift-right: [w167] -> _
    shift-left: "Source/Drain\nRange mode" -> [w172]
    shift-right: [w168] -> _
    shift-left: "Gate Range" -> [w173]
    shift-right: [w169] -> _
    shift-left: "Gate Range\nmode" -> [w174]
    shift-right: [w170] -> _
    shift-left: "Gate: Compliance" -> [w183]
    shift-right: [w179] -> _
    shift-left: "Drain: Compliance" -> [w184]
    shift-right: [w180] -> _
    shift-left: w50 -> [w185]
    shift-right: [w181] -> w17
    shift-left: w24 -> [w186]
    shift-right: [w66] -> w26
    shift-left: w51 -> [w187]
    shift-right: [w182] -> _
    shift-left: w14 -> [w188]
    shift-right: [w69] -> _
    tunnel: "Panel Controls 2" -> [w165]
    shift-right: [w81] -> _
    shift-left: w22 -> [w164]
    shift-right: [w117] -> _
    shift-left: i32[] [] -> [w160]
    tunnel: w31 -> [w159] mode=indexing
    shift-right: [w80] -> _
    shift-left: w22 -> [w136]
    shift-right: [w111] -> _
    shift-left: w20 -> [w122]
    shift-right: [w112] -> _
    shift-left: w18 -> [w114]
    shift-right: [w74] -> _
    shift-left: w22 -> [w102]
    shift-right: [w75] -> _
    shift-left: w22 -> [w101]
    shift-right: [w79] -> _
    shift-left: w22 -> [w90]
    shift-right: [w78] -> _
    shift-left: w22 -> [w89]
    shift-right: [w72] -> _
    shift-left: w22 -> [w88]
    shift-right: [w82] -> _
    shift-left: w22 -> [w87]
    shift-right: [w73] -> _
    shift-left: w22 -> [w86]
    shift-right: [w71] -> _
    shift-left: w22 -> [w85]
    shift-right: [w77] -> _
    shift-left: w22 -> [w84]
    shift-right: [w76] -> _
    shift-left: w22 -> [w83]
    i -> [w125]
    stop <- "Interrupt program" stop-if-true
    # "Is off"
    # "Is on"
    # "Ig off"
    # "Ig on"
    # "Is min"
    # "Is max"
    # "Ig min"
    # "Ig max"
    # "Id min"
    # "Id max"
    # "Id off"
    # "Id on"
    # "Filepath and name"
    # "Limit of command arguments (array columns). Raise if needed."
    # "Serial port data (string)"
    # "Serial port data (table)"
    # "Serial port data"
    # "For loop counter"
    # "<-----Equivalent to the 4155C \"Write\" subvi.----->"
    # "Headers"
    # "Save transfer curves in file."
    # "Filepath and name"
    # "Save time-dependent data."
    # "Use the time offset if your measurements do not start at t=0."
    # "Time for Imax, Imin, Ion, Ioff"
    # "Rest of elements of command"
    # "First element of command\n(case select)"
    n20 = Add(x=w125, y=1) -> (x+y=→"Line running":i32)
    n21 = Add(x=w130, y=1) -> (x+y=→"Total lines":i32)
    n22 = Index Array(array=w159, index=0 ("line index")) -> (element=w154:string)
    "Command running:" <- w154
    n23 = control-ref of="Interrupt scan"() -> (w178:refnum<vi>)
    n24 = Spreadsheet String To Array(delimiter (Tab)=" ", format string="%s", spreadsheet string=w154, array type (2D Dbl)=string[] []) -> (array=w152:string[])
    n25 = Delete From Array(array=w152, index=0) -> (deleted portion=w103:string, array with subset deleted=w151:string[])  [unwired: 1 in]
    n26 = call "Elapsed Time"("Reset"="Reset", "Auto Reset"="Auto Reset") -> ("Elapsed Time (s)"=w161:dbl)  [unwired: 10 in, 7 out]
    n27 = case shown="2" "Time Units" {
      tunnel: ["-sec" "-min" "-h"] -> w162
      tunnel: [w192 w196 w199] -> w132
      tunnel: w161 -> [w192 w195 w200]
      frame 0, Default {
      }
      frame 1 {
        n28 = Divide(x=w195, y=60.0) -> (x/y=w196:dbl)
      }
      frame 2 {
        n29 = Divide(x=w200, y=3600.0) -> (x/y=w199:dbl)
      }
    }
    n30 = Add(x=w132, y="Time Offset") -> (x+y=w131:dbl)
    n31 = To Long Integer(number=w131) -> (32bit integer=w116:i32)
    "Elapsed Time" <- w116
    n32 = case shown="\"sample-fpp\"" w103 {
      tunnel: w151 -> [w231 w263 w294 w388 w494 w629 w744 w899 w926 w994 w1034 w1072 w1106 w1133 _ _ w1276 w1350 _ w1441 w1498 w1553 w1636 w1711 w1744]
      tunnel: w188 -> [w226 w259 w292 w395 w554 w637 w751 w907 w943 w983 w1026 w1065 w1100 w1126 w1158 w1213 w1254 w1332 w1376 w1428 w1485 w1541 w1630 w1707 w1746]
      tunnel: w187 -> [w225 w258 w283 w366 w539 w606 w722 w875 w944 w984 w1027 w1066 w1101 w1127 w1163 w1215 w1282 w1356 w1380 w1447 w1504 w1559 w1642 w1665 w1750]
      tunnel: w186 -> [w224 w257 w282 w365 w538 w605 w721 w872 w945 w985 w1028 w1067 w1102 w1128 w1162 w1186 w1281 w1355 w1379 w1446 w1503 w1558 w1641 w1664 w1749]
      tunnel: w185 -> [w223 w256 w291 w391 w514 w633 w747 w903 w953 w993 w1025 w1064 w1099 w1125 w1161 w1210 w1245 w1324 w1385 w1421 w1478 w1534 w1629 w1706 w1751]
      tunnel: w184 -> [w222 w255 w290 w393 w552 w635 w749 w905 w952 w992 w1033 w1071 w1105 w1132 w1160 w1195 w1280 w1354 w1388 w1445 w1502 w1557 w1640 w1715 w1752]
      tunnel: w183 -> [w221 w254 w289 w392 w551 w634 w748 w904 w951 w991 w1032 w1070 w1104 w1131 w1159 w1196 w1255 w1333 w1387 w1429 w1486 w1542 w1631 w1708 w1754]
      tunnel: [w225 w258 w281 w390 w549 w631 w746 w901 w944 w984 w1027 w1066 w1101 w1127 w1163 w1215 w1246 w1306 w1378 w1422 w1479 w1535 w1582 w1667 w1750] -> w182
      tunnel: [w224 w257 w280 w389 w548 w630 w745 w900 w945 w985 w1028 w1067 w1102 w1128 w1162 w1185 w1256 w1307 w1377 w1430 w1487 w1543 w1581 w1666 w1748] -> w115
      tunnel: [w223 w256 w291 w391 w510 w633 w747 w903 w946 w986 w1025 w1064 w1099 w1125 w1161 w1210 w1245 w1324 w1385 w1421 w1478 w1534 w1629 w1706 w1751] -> w181
      tunnel: [w222 w255 w290 w393 w552 w635 w749 w905 w952 w992 w1033 w1071 w1105 w1132 w1160 w1195 w1280 w1354 w1388 w1445 w1502 w1557 w1640 w1715 w1752] -> w180
      tunnel: [w221 w254 w289 w392 w551 w634 w748 w904 w951 w991 w1032 w1070 w1104 w1131 w1159 w1196 w1255 w1333 w1387 w1429 w1486 w1542 w1631 w1708 w1754] -> w179
      tunnel: [w226 w259 w292 w395 w554 w637 w751 w907 w943 w983 w1026 w1065 w1100 w1126 w1158 w1213 w1254 w1332 w1376 w1428 w1485 w1541 w1630 w1707 w1746] -> w69
      tunnel: w178 -> [_ _ _ w397 w558 w642 w753 w911 _ _ _ _ _ _ _ _ w1251 w1329 _ w1427 w1484 w1540 w1602 w1683 _]
      tunnel: "Gate" -> [_ _ _ w375 w542 w616 w731 w886 _ _ _ _ _ _ _ _ _ _ _ _ _ _ _ _ _]
      tunnel: "Drain 2" -> [_ _ _ w374 w541 w615 w730 w885 _ _ _ _ _ _ _ _ _ _ _ _ _ _ _ _ _]
      tunnel: "Panel Controls" -> [_ _ _ _ _ w614 w656 w884 _ _ _ _ _ _ _ _ _ _ _ _ _ _ _ _ _]
      tunnel: w174 -> [w220 w253 w288 w359 w532 w599 w715 w870 w950 w990 _ w1063 w1098 w1124 w1157 w1197 w1241 w1320 w1381 w1417 w1474 w1530 w1625 w1702 w1755]
      tunnel: w173 -> [w219 w252 w287 w358 w531 w598 w714 w869 w949 w989 w1031 _ w1089 w1130 w1156 w1198 w1242 w1321 w1382 w1418 w1475 w1531 w1626 w1703 w1756]
      tunnel: w172 -> [w218 w251 w286 w357 w530 w597 w713 w868 w948 w988 w1030 w1069 w1103 _ w1155 w1199 w1243 w1322 w1383 w1419 w1476 w1532 w1627 w1704 w1757]
      tunnel: w171 -> [w217 w250 w285 w356 w529 w596 w712 w871 w947 w987 w1029 w1068 _ w1129 w1154 w1200 w1244 w1323 w1384 w1420 w1477 w1533 w1628 w1705 w1758]
      tunnel: [w220 w253 w288 w359 w532 w599 w715 w870 w950 w990 w1024 w1063 w1098 w1124 w1157 w1197 w1241 w1320 w1381 w1417 w1474 w1530 w1625 w1702 w1755] -> w170
      tunnel: [w219 w252 w287 w358 w531 w598 w714 w869 w949 w989 w1031 w1055 w1089 w1130 w1156 w1198 w1242 w1321 w1382 w1418 w1475 w1531 w1626 w1703 w1756] -> w169
      tunnel: [w218 w251 w286 w357 w530 w597 w713 w868 w948 w988 w1030 w1069 w1103 w1123 w1155 w1199 w1243 w1322 w1383 w1419 w1476 w1532 w1627 w1704 w1757] -> w168
      tunnel: [w217 w250 w285 w356 w529 w596 w712 w871 w947 w987 w1029 w1068 w1090 w1129 w1154 w1200 w1244 w1323 w1384 w1420 w1477 w1533 w1628 w1705 w1758] -> w167
      tunnel: w166 -> [_ _ _ w351 w526 _ w707 _ _ _ _ _ _ _ _ _ _ _ _ _ _ _ _ _ _]
      tunnel: w165 -> [_ _ _ w349 w525 _ _ _ _ _ _ _ _ _ _ _ _ _ _ _ _ _ _ _ _]
      tunnel: [w216 w246 w278 w311 w502 w586 w668 w857 w942 w981 w1023 w1054 w1088 w1122 w1153 w1181 w1233 w1290 w1375 w1406 w1467 w1524 w1579 w1660 w1747] -> w81
      tunnel: w164 -> [w216 w246 w278 w346 w502 w586 w703 w857 w942 w981 w1023 w1054 w1088 w1122 w1153 w1181 w1233 w1290 w1375 w1406 w1467 w1524 w1579 w1660 w1747]
      tunnel: w131 -> [_ _ _ w345 w499 w584 w702 w854 _ _ _ _ _ _ _ w1179 w1231 w1302 _ w1403 w1464 w1521 w1576 w1656 _]
      tunnel: w162 -> [_ _ _ w342 w498 w582 w699 w853 _ _ _ _ _ _ _ w1177 w1229 w1301 _ w1402 w1463 w1520 w1575 w1657 _]
      tunnel: w116 -> [_ _ _ w338 _ _ w695 _ _ _ _ _ _ _ _ _ _ _ _ _ _ _ _ _ _]
      tunnel: [w215 w245 w277 w315 w501 w585 w672 w856 w941 w980 w1022 w1053 w1087 w1121 w1152 w1180 w1232 w1304 w1374 w1405 w1466 w1523 w1578 w1659 w1753] -> w117
      tunnel: w160 -> [w215 w245 w277 w341 w501 w585 w698 w856 w941 w980 w1022 w1053 w1087 w1121 w1152 w1180 w1232 w1304 w1374 w1405 w1466 w1523 w1578 w1659 w1753]
      tunnel: [w214 w244 w276 w310 w497 w581 w667 w852 w940 w979 w1021 w1052 w1086 w1120 w1151 w1176 w1228 w1289 w1373 w1401 w1462 w1519 w1574 w1655 w1742] -> w80
      tunnel: w136 -> [w214 w244 w276 w337 w497 w581 w694 w852 w940 w979 w1021 w1052 w1086 w1120 w1151 w1176 w1228 w1289 w1373 w1401 w1462 w1519 w1574 w1655 w1742]
      tunnel: [w213 w243 w275 w330 w496 w580 w687 w851 w939 w978 w1020 w1051 w1085 w1119 w1150 w1175 w1227 w1300 w1372 w1400 w1461 w1518 w1573 w1654 w1741] -> w111
      tunnel: w122 -> [w213 w243 w275 w330 w496 w580 w687 w851 w939 w978 w1020 w1051 w1085 w1119 w1150 w1175 w1227 w1300 w1372 w1400 w1461 w1518 w1573 w1654 w1740]
      tunnel: w116 -> [_ _ _ _ _ _ _ _ _ _ _ _ _ _ _ _ _ _ _ _ _ _ _ _ _]
      tunnel: [w212 w242 w274 w329 w495 w579 w686 w850 w938 w977 w1019 w1050 w1084 w1118 w1149 w1174 w1226 w1299 w1371 w1399 w1460 w1517 w1572 w1653 w1726] -> w112
      tunnel: w114 -> [w212 w242 w274 w329 w495 w579 w686 w850 w938 w977 w1019 w1050 w1084 w1118 w1149 w1174 w1226 w1299 w1371 w1399 w1460 w1517 w1572 w1653 w1726]
      tunnel: [w210 w240 w272 w304 w492 w577 w661 w848 w936 w976 w1018 w1048 w1082 w1116 w1147 w1172 w1225 w1298 w1370 w1398 w1459 w1515 w1571 w1652 w1725] -> w74
      tunnel: w102 -> [w210 w240 w272 w328 w492 w577 w685 w848 w936 w976 w1018 w1048 w1082 w1116 w1147 w1172 w1225 w1298 w1370 w1398 w1459 w1515 w1571 w1652 w1725]
      tunnel: [w211 w241 w273 w305 w493 w578 w662 w849 w937 w975 w1017 w1049 w1083 w1117 w1148 w1173 w1224 w1297 w1369 w1397 w1458 w1516 w1570 w1651 w1724] -> w75
      tunnel: w101 -> [w211 w241 w273 w327 w493 w578 w684 w849 w937 w975 w1017 w1049 w1083 w1117 w1148 w1173 w1224 w1297 w1369 w1397 w1458 w1516 w1570 w1651 w1724]
      tunnel: [w203 w233 w265 w309 w489 w575 w666 w846 w929 w973 w1015 w1046 w1080 w1114 w1145 w1165 w1217 w1288 w1368 w1390 w1451 w1508 w1563 w1646 w1717] -> w79
      tunnel: w90 -> [w203 w233 w265 w323 w489 w575 w680 w846 w929 w973 w1015 w1046 w1080 w1114 w1145 w1165 w1217 w1288 w1368 w1390 w1451 w1508 w1563 w1646 w1717]
      tunnel: [w202 w232 w264 w308 w490 w576 w665 w847 w928 w974 w1016 w1047 w1081 w1115 w1146 w1164 w1216 w1287 w1367 w1389 w1450 w1507 w1562 w1645 w1716] -> w78
      tunnel: w89 -> [w202 w232 w264 w322 w490 w576 w679 w847 w928 w974 w1016 w1047 w1081 w1115 w1146 w1164 w1216 w1287 w1367 w1389 w1450 w1507 w1562 w1645 w1716]
      tunnel: [w205 w235 w267 w314 w488 w573 w671 w844 w934 w971 w1013 w1044 w1078 w1112 w1143 w1167 w1219 w1292 w1362 w1392 w1453 w1510 w1565 w1644 w1721] -> w72
      tunnel: w88 -> [w205 w235 w267 w321 w488 w573 w678 w844 w934 w971 w1013 w1044 w1078 w1112 w1143 w1167 w1219 w1292 w1362 w1392 w1453 w1510 w1565 w1644 w1721]
      tunnel: [w204 w234 w266 w312 w491 w574 w669 w845 w935 w972 w1014 w1045 w1079 w1113 w1144 w1166 w1218 w1291 w1361 w1391 w1452 w1509 w1564 w1643 w1720] -> w82
      tunnel: w87 -> [w204 w234 w266 w320 w491 w574 w677 w845 w935 w972 w1014 w1045 w1079 w1113 w1144 w1166 w1218 w1291 w1361 w1391 w1452 w1509 w1564 w1643 w1720]
      tunnel: [w207 w237 w269 w303 w487 w571 w660 w842 w932 w969 w1011 w1042 w1076 w1110 w1141 w1169 w1221 w1294 w1364 w1394 w1455 w1512 w1567 w1648 w1723] -> w73
      tunnel: w86 -> [w207 w237 w269 w319 w487 w571 w676 w842 w932 w969 w1011 w1042 w1076 w1110 w1141 w1169 w1221 w1294 w1364 w1394 w1455 w1512 w1567 w1648 w1723]
      tunnel: [w206 w236 w268 w302 w486 w572 w659 w843 w933 w970 w1012 w1043 w1077 w1111 w1142 w1168 w1220 w1293 w1363 w1393 w1454 w1511 w1566 w1647 w1722] -> w71
      tunnel: w85 -> [w206 w236 w268 w318 w486 w572 w675 w843 w933 w970 w1012 w1043 w1077 w1111 w1142 w1168 w1220 w1293 w1363 w1393 w1454 w1511 w1566 w1647 w1722]
      tunnel: [w209 w239 w271 w307 w485 w569 w664 w840 w930 w967 w1009 w1040 w1074 w1108 w1139 w1171 w1223 w1296 w1366 w1396 w1457 w1514 w1569 w1650 w1719] -> w77
      tunnel: w84 -> [w209 w239 w271 w317 w485 w569 w674 w840 w930 w967 w1009 w1040 w1074 w1108 w1139 w1171 w1223 w1296 w1366 w1396 w1457 w1514 w1569 w1650 w1719]
      tunnel: [w208 w238 w270 w306 w484 w570 w663 w841 w931 w968 w1010 w1041 w1075 w1109 w1140 w1170 w1222 w1295 w1365 w1395 w1456 w1513 w1568 w1649 w1718] -> w76
      tunnel: w83 -> [w208 w238 w270 w316 w484 w570 w673 w841 w931 w968 w1010 w1041 w1075 w1109 w1140 w1170 w1222 w1295 w1365 w1395 w1456 w1513 w1568 w1649 w1718]
      frame "wait" {
        n33 = Index Array(array=w231, index=0 ("Index")) -> (element=w229:string)
        n34 = Decimal String To Number(string=w229, default (0L)=u32 0) -> (number=w228:u32)  [unwired: 1 in, 1 out]
        n35 = Wait (ms)(milliseconds to wait=w228) -> ()  [unwired: 1 out]
      }
      frame "wait-min" {
        n36 = Index Array(array=w263, index=0 ("Index")) -> (element=w261:string)
        n37 = Decimal String To Number(string=w261, default (0L)=u32 0) -> (number=w249:u32)  [unwired: 1 in, 1 out]
        n38 = Multiply(x=w249, y=u32 60000) -> (x*y=w248:u32)
        n39 = Wait (ms)(milliseconds to wait=w248) -> ()  [unwired: 1 out]
      }
      frame "standby" {
        n40 = Index Array(array=w294, index=0 ("Index")) -> (element=w284:string)
        n41 = case shown="\"off\", Default" w284 {
          tunnel: [":PAGE:SCON:STAN 0" ":PAGE:SCON:STAN 1"] -> w279
          frame "off", Default {
          }
          frame "on" {
          }
        }
        n42 = VISA Write(VISA resource name=w283, write buffer=w279, error in (no error)=w282) -> (VISA resource name out=w281:refnum<visa-resource-name>, error out=w280:errorcluster)  [unwired: 1 out]
      }
      frame "transfer" {
        # "Is off"
        # "Is on"
        # "Ig off"
        # "Ig on"
        # "Is min"
        # "Is max"
        # "Ig min"
        # "Ig max"
        # "Id min"
        # "Id max"
        # "Id off"
        # "Id on"
        n43 = Delete From Array(array=w388, index=0 ("Index")) -> (deleted portion=w386:string, array with subset deleted=w385:string[])  [unwired: 1 in]
        n44 = Bundle By Name(cluster=w349, "Emergency Stop"=w397) -> (w350:T2)
        n45 = Number To Decimal String(number=w345) -> (decimal integer string=w344:string)  [unwired: 1 in]
        n46 = case shown="\"d\", Default" w386 {
          tunnel: [w482 w483] -> w384
          frame "s" {
            w482 = u16 0 items=["Single", "Double"] ("sweep mode")
          }
          frame "d", Default {
            w483 = u16 1 items=["Single", "Double"] ("sweep mode")
          }
        }
        n47 = Fract/Exp String To Number(string=w385) -> (number=w370:dbl[])  [unwired: 3 in, 1 out]
        n48 = Concatenate Strings(w395, "-transfer-" ("Prefix"), w344, w342, ".txt" ("Suffix (transfer)")) -> (w396:string)
        n49 = VISA Write(VISA resource name=w366, write buffer=":PAGE:CHAN:MODE SWE;" ("write buffer (\"\")"), error in (no error)=w365) -> (VISA resource name out=w363:refnum<visa-resource-name>, error out=w364:errorcluster)  [unwired: 1 out]
        n50 = local read "Plot transfer curve extrema vs time"() -> (w297:bool)
        n51 = String To Path(string=w396) -> (path=w394:path)
        n52 = Index Array(array=w370, index #1=0 ("Index")) -> (element #1=w383:dbl, element #2=w382:dbl, element #3=w381:dbl)  [unwired: 2 in]
        n53 = Delete From Array(array=w370, length=3 ("Length"), index=0 ("Index")) -> (array with subset deleted=w368:dbl[])  [unwired: 1 out]
        n54 = case shown="True" w297 {
          tunnel: w341 -> [w399 w402]
          tunnel: w338 -> [_ w401]
          tunnel: [w399 w400] -> w315
          frame False {
          }
          frame True {
            n55 = Build Array (concatenate)(w402, w401) -> (w400:i32[])
          }
        }
        n56 = Bundle By Name(cluster=w375, "Gate Start"=w383, "Gate Stop"=w382, "Gate Step (linear only)"=w381, "Gate Compliance"=w392, "Range mode"=w359, "Range"=w358) -> (w360:T6)
        n57 = Index Array(array=w368, index #1=0 ("Index")) -> (element #1=w378:dbl, element #2=w377:dbl, element #3=w376:dbl)  [unwired: 2 in]
        n58 = call <vilib>:"compatOverwrite.vi"("overwrite (F)"=TRUE) -> ("overwrite?"=w348:T8)
        n59 = Bundle By Name(cluster=w374, "Drain Start"=w378, "Drain Stop"=w377, "Drain Step"=w376, "Drain Compliance"=w393, "Range mode"=w357, "Range"=w356) -> (w361:T7)
        n60 = call "4155C Transfer.vi"("VISA resource name in"=w363, "Gate"=w360, "Drain"=w361, "Timings"=w391, "error in (no error)"=w364, "SMU4"=w351, "sweep mode"=w384, "Panel Controls"=w350) -> ("VG"=w347:dbl[], "Outparams"=w355:T9, "VISA Resource Name out"=w390:refnum<visa-resource-name>, "IS"=w325:dbl[], "ID"=w326:dbl[], "IG"=w324:dbl[], "error out"=w339:errorcluster, "SMU4"=w352:dbl[])  [unwired: 12 in]
        n61 = Unbundle By Name(w355) -> ("V2 Step"=w354:dbl, "V2 Start"=w353:dbl, "Number of points"=w313:i32)
        n62 = call "4155C Split array.vi"("Number of VAR2 steps"=w313, "Y2 data in"=w326, "X data in"=w347, "Y1 data in"=w325, "Y3 data in"=w324, "error in (no error)"=w339) -> ("Array of clusters"=w340:cluster{"Y data in":dbl[], "X data in":dbl[]}[], "error out"=w301:errorcluster)  [unwired: 1 in]
        n63 = case shown="True" "Plot transfer curve extrema vs time" {
          tunnel: w346 -> [w405 w481]
          tunnel: w337 -> [w406 w476]
          tunnel: w328 -> [w412 w472]
          tunnel: w327 -> [w413 w471]
          tunnel: w326 -> [_ w468]
          tunnel: w325 -> [_ w466]
          tunnel: w324 -> [_ w465]
          tunnel: w323 -> [w407 w461]
          tunnel: w322 -> [w409 w460]
          tunnel: w321 -> [w403 w457]
          tunnel: w320 -> [w404 w456]
          tunnel: w319 -> [w411 w453]
          tunnel: w318 -> [w410 w452]
          tunnel: w317 -> [w415 w449]
          tunnel: w316 -> [w414 w448]
          tunnel: w315 -> [_ w441]
          tunnel: [w403 w436] -> w314
          tunnel: w313 -> [_ w435]
          tunnel: [w404 w434] -> w312
          tunnel: [w405 w433] -> w311
          tunnel: [w406 w432] -> w310
          tunnel: [w407 w431] -> w309
          tunnel: [w409 w430] -> w308
          tunnel: [w415 w429] -> w307
          tunnel: [w414 w428] -> w306
          tunnel: [w413 w427] -> w305
          tunnel: [w412 w426] -> w304
          tunnel: [w411 w425] -> w303
          tunnel: [w410 w424] -> w302
          tunnel: w301 -> [w408 w423]
          tunnel: [w408 w419] -> w300
          frame False {
          }
          frame True {
            # "Adjusts graph colors."
            # "Adjusts graph colors."
            # "Ion will be the middle element of the array. The calculation of the index is done only once, since Is, Id, and Ig have the same dimensions."
            # "abs(Ig)"
            # "abs(Is)"
            # "Y1: Is\nY2: Id\nY3: Ig"
            # "abs(Id)"
            # "Adjusts graph colors."
            # "Adjusts graph colors."
            # "Adjusts graph colors."
            n64 = Absolute Value(x=w466) -> (abs(x)=w451:dbl[])
            n65 = Absolute Value(x=w468) -> (abs(x)=w467:dbl[])
            n66 = Absolute Value(x=w465) -> (abs(x)=w454:dbl[])
            n67 = Array Size(array=w467) -> (size(s)=w475:i32)
            n68 = Divide(x=w475, y=2) -> (x/y=w418:dbl)
            n69 = Subtract(x=w418, y=1) -> (x-y=w417:dbl)
            n70 = Array Max & Min(array=w451) -> (max value=w458:dbl, min value=w459:dbl)  [unwired: 2 out]
            n71 = Array Max & Min(array=w467) -> (max value=w480:dbl, min value=w464:dbl)  [unwired: 2 out]
            n72 = Array Max & Min(array=w454) -> (max value=w463:dbl, min value=w462:dbl)  [unwired: 2 out]
            n73 = Index Array(array=w451, index=w417) -> (element=w442:dbl)
            n74 = Index Array(array=w451, index=0) -> (element=w443:dbl)
            n75 = Index Array(array=w467, index=w417) -> (element=w444:dbl)
            n76 = Index Array(array=w467, index=0) -> (element=w445:dbl)
            n77 = Index Array(array=w454, index=w417) -> (element=w447:dbl)
            n78 = Index Array(array=w454, index=0) -> (element=w446:dbl)
            n79 = local write "Ig max"(w463) -> ()
            n80 = local write "Ig min"(w462) -> ()
            n81 = local write "Is max"(w458) -> ()
            n82 = local write "Is min"(w459) -> ()
            n83 = local write "Id max"(w480) -> ()
            n84 = local write "Id min"(w464) -> ()
            n85 = Build Array (concatenate)(w457, w458) -> (w436:dbl[])
            n86 = Build Array (concatenate)(w456, w459) -> (w434:dbl[])
            n87 = local write "Is off"(w443) -> ()
            n88 = local write "Is on"(w442) -> ()
            n89 = Build Array (concatenate)(w481, w480) -> (w433:dbl[])
            n90 = Build Array (concatenate)(w476, w464) -> (w432:dbl[])
            n91 = Build Array (concatenate)(w461, w463) -> (w431:dbl[])
            n92 = Build Array (concatenate)(w460, w462) -> (w430:dbl[])
            n93 = Build Array (concatenate)(w449, w442) -> (w429:dbl[])
            n94 = Build Array (concatenate)(w448, w443) -> (w428:dbl[])
            n95 = Build Array (concatenate)(w471, w444) -> (w427:dbl[])
            n96 = Build Array (concatenate)(w472, w445) -> (w426:dbl[])
            n97 = Build Array (concatenate)(w453, w447) -> (w425:dbl[])
            n98 = Build Array (concatenate)(w452, w446) -> (w424:dbl[])
            n99 = local write "Ig off"(w446) -> ()
            n100 = local write "Ig on"(w447) -> ()
            n101 = local write "Id off"(w445) -> ()
            n102 = local write "Id on"(w444) -> ()
            n103 = control-ref of="Imax vs time"() -> (w470:refnum<vi>)
            n104 = control-ref of="Imin vs time"() -> (w469:refnum<vi>)
            n105 = control-ref of="Ion vs time"() -> (w438:refnum<vi>)
            n106 = control-ref of="Ioff vs time"() -> (w437:refnum<vi>)
            n107 = control-ref of="I vs Vg"() -> (w479:refnum<vi>)
            n108 = call "4155C Split array.vi"("Number of VAR2 steps"=w435, "Y2 data in"=w427, "X data in"=w441, "Y1 data in"=w429, "Y3 data in"=w425, "error in (no error)"=w423) -> ("Array of clusters"=w439:cluster{"Y data in":dbl[], "X data in":dbl[]}[], "error out"=w422:errorcluster)  [unwired: 1 in]
            n109 = call "4155C Split array.vi"("Number of VAR2 steps"=w435, "Y2 data in"=w426, "X data in"=w441, "Y1 data in"=w428, "Y3 data in"=w424, "error in (no error)"=w422) -> ("Array of clusters"=w440:cluster{"Y data in":dbl[], "X data in":dbl[]}[], "error out"=w421:errorcluster)  [unwired: 1 in]
            n110 = call "4155C Split array.vi"("Number of VAR2 steps"=w435, "Y2 data in"=w433, "X data in"=w441, "Y1 data in"=w436, "Y3 data in"=w431, "error in (no error)"=w421) -> ("Array of clusters"=w478:cluster{"Y data in":dbl[], "X data in":dbl[]}[], "error out"=w420:errorcluster)  [unwired: 1 in]
            n111 = call "4155C Split array.vi"("Number of VAR2 steps"=w435, "Y2 data in"=w432, "X data in"=w441, "Y1 data in"=w434, "Y3 data in"=w430, "error in (no error)"=w420) -> ("Array of clusters"=w477:cluster{"Y data in":dbl[], "X data in":dbl[]}[], "error out"=w419:errorcluster)  [unwired: 1 in]
            n112 = call "4155C Config Chart Colours.vi"("Numeric"=w435, "XY Graph 2"=w470) -> ()  [unwired: 6 in]
            n113 = call "4155C Config Chart Colours.vi"("Numeric"=w435, "XY Graph 2"=w469) -> ()  [unwired: 6 in]
            n114 = call "4155C Config Chart Colours.vi"("Numeric"=w435, "XY Graph 2"=w438) -> ()  [unwired: 6 in]
            n115 = call "4155C Config Chart Colours.vi"("Numeric"=w435, "XY Graph 2"=w437) -> ()  [unwired: 6 in]
            n116 = call "4155C Config Chart Colours.vi"("Numeric"=w435, "XY Graph 2"=w479) -> ()  [unwired: 6 in]
            n117 = local write "Imax vs time"(w478) -> ()
            n118 = local write "Imin vs time"(w477) -> ()
            n119 = local write "Ion vs time"(w439) -> ()
            n120 = local write "Ioff vs time"(w440) -> ()
          }
        }
        n121 = local write "I vs Vg"(w340) -> ()
        n122 = Open/Create/Replace File(file path (use dialog)=w394, error in=w300, operation (0:open)=w348) -> (refnum out=w335:refnum<file>, error out=w333:errorcluster)  [unwired: 3 in, 1 out]
        n123 = call "4155C Make Big 2d array.vi"("1D Var1"=w347, "1d IS"=w325, "1d ID"=w326, "1d IG"=w324, "1d SMU4"=w352, "SMU4"=w351, "VAR2 START"=w353, "Number of VAR2 steps"=w313, "VAR2 STEP"=w354, "VAR1 Name"="Vg", "Decimal places in header"=i8 1, "VAR2 Name"="Vd") -> ("Header array"=w336:string[], "Data array"=w334:dbl[][])  [unwired: 14 in]
        n124 = call "4155C Write array to file.vi"("Byte Stream File Refnum"=w335, "Header"=w336, "Data Array"=w334, "error in (no error)"=w333) -> ("dup refnum"=w332:refnum<file>, "error out"=w331:errorcluster)  [unwired: 1 in]
        n125 = Close File(refnum=w332, error in=w331) -> (error out=w389:errorcluster)  [unwired: 1 out]
      }
      frame "pulsedstressV" {
        w508 = 0
        n126 = Number To Decimal String(number=w499) -> (decimal integer string=w555:string)  [unwired: 1 in]
        n127 = Delete From Array(array=w494, index=0 ("Index")) -> (deleted portion=w546:string, array with subset deleted=w545:string[])  [unwired: 1 in]
        n128 = Bundle By Name(cluster=w525, "Emergency Stop"=w558) -> (w527:T2)
        n129 = VISA Write(VISA resource name=w539, write buffer=":PAGE:CHAN:MODE SWE;" ("write buffer (\"\")"), error in (no error)=w538) -> (VISA resource name out=w536:refnum<visa-resource-name>, error out=w537:errorcluster)  [unwired: 1 out]
        n130 = Concatenate Strings(w554, "-pulsedstressV-" ("Substring"), w555, w498, ".txt" ("Substring")) -> (w557:string)
        n131 = case shown="\"d\", Default" w546 {
          tunnel: [w567 w568] -> w544
          frame "s" {
            w567 = u16 0 items=["Single", "Double"] ("sweep mode")
          }
          frame "d", Default {
            w568 = u16 1 items=["Single", "Double"] ("sweep mode")
          }
        }
        n132 = Fract/Exp String To Number(string=w545) -> (number=w540:dbl[])  [unwired: 3 in, 1 out]
        n133 = String To Path(string=w557) -> (path=w553:path)
        n134 = Index Array(array=w540, index #1=0 ("Index")) -> (element #1=w517:dbl, element #2=w516:dbl, element #3=w513:dbl, element #4=w512:dbl, element #5=w511:dbl, element #6=w515:dbl)  [unwired: 5 in]
        n135 = Bundle By Name(cluster=w514, "Pulse period"=w512, "Base voltage"=w513, "Pulse width"=w511) -> (w510:T4)
        n136 = Unbundle By Name(w510) -> ("Pulse period"=w518:dbl)
        n137 = Bundle By Name(cluster=w542, "Gate Start"=w516, "Gate Stop"=w517, "Gate Step (linear only)"=0, "Gate Compliance"=w551, "Range mode"=w532, "Range"=w531) -> (w533:T6)
        n138 = call <vilib>:"compatOverwrite.vi"("overwrite (F)"=TRUE) -> ("overwrite?"=w503:T8)
        n139 = Bundle By Name(cluster=w541, "Drain Start"=w515, "Drain Stop"=w508, "Drain Step"=w508, "Drain Compliance"=w552, "Range mode"=w530, "Range"=w529) -> (w534:T7)
        n140 = call "4155C PulsedStressV.vi"("VISA resource name in"=w536, "sweep mode"=w544, "Panel Controls"=w527, "Gate"=w533, "Drain"=w534, "Timings"=w510, "error in (no error)"=w537, "SMU4"=w526) -> ("VISA Resource Name out"=w549:refnum<visa-resource-name>, "ID"=w506:dbl[], "IG"=w504:dbl[], "Outparams"=w528:T9, "error out"=w550:errorcluster)  [unwired: 3 in]
        n141 = Unbundle By Name(w528) -> ("Number of points"=w505:i32)  [unwired: 2 out]
        n142 = for {
          N: w505 -> [_]
          tunnel: [w564] -> w507 mode=indexing
          tunnel: w518 -> [w566]
          i -> [w565]
          n143 = Multiply(x=w566, y=w565) -> (x*y=w564:dbl)
        }
        n144 = Insert Into Array(array=dbl[][] [] ("Input Array"), new element=w507) -> (w519:dbl[][])  [unwired: 2 in]
        n145 = Insert Into Array(array=w519, new element=w506) -> (w524:dbl[][])  [unwired: 2 in]
        n146 = Insert Into Array(array=w524, new element=w504) -> (w523:dbl[][])  [unwired: 2 in]
        n147 = Transpose 2D Array(2D array=w523) -> (transposed array=w522:dbl[][])
        n148 = Open/Create/Replace File(file path (use dialog)=w553, error in=w550, operation (0:open)=w503) -> (refnum out=w561:refnum<file>, error out=w562:errorcluster)  [unwired: 3 in, 1 out]
        n149 = call "4155C Write array to file.vi"("Byte Stream File Refnum"=w561, "Header"=string[] ["Time /s", "Id /A", "Ig /A"], "Data Array"=w522, "error in (no error)"=w562) -> ("dup refnum"=w559:refnum<file>, "error out"=w560:errorcluster)  [unwired: 1 in]
        n150 = Close File(refnum=w559, error in=w560) -> (error out=w548:errorcluster)  [unwired: 1 out]
      }
      frame "transfer-fpp" {
        n151 = Number To Decimal String(number=w584) -> (decimal integer string=w638:string)  [unwired: 1 in]
        n152 = Bundle By Name(cluster=w614, "Emergency Stop"=w642) -> (w650:T1)
        n153 = Delete From Array(array=w629, index=0 ("Index")) -> (deleted portion=w627:string, array with subset deleted=w626:string[])  [unwired: 1 in]
        n154 = Concatenate Strings(w637, "-transferfpp-" ("Substring"), w638, w582, ".txt" ("Substring")) -> (w640:string)
        n155 = VISA Write(VISA resource name=w606, write buffer=":PAGE:CHAN:MODE SWE;" ("write buffer (\"\")"), error in (no error)=w605) -> (VISA resource name out=w603:refnum<visa-resource-name>, error out=w604:errorcluster)  [unwired: 1 out]
        n156 = case shown="\"d\", Default" w627 {
          tunnel: [w651 w652] -> w625
          frame "s" {
            w651 = u16 0 items=["Single", "Double"] ("sweep mode")
          }
          frame "d", Default {
            w652 = u16 1 items=["Single", "Double"] ("sweep mode")
          }
        }
        n157 = Fract/Exp String To Number(string=w626) -> (number=w610:dbl[])  [unwired: 3 in, 1 out]
        n158 = String To Path(string=w640) -> (path=w636:path)
        n159 = Index Array(array=w610, index #1=0 ("Index")) -> (element #1=w624:dbl, element #2=w623:dbl, element #3=w622:dbl)  [unwired: 2 in]
        n160 = Delete From Array(array=w610, length=3 ("Length"), index=0 ("Index")) -> (array with subset deleted=w608:dbl[])  [unwired: 1 out]
        n161 = Bundle By Name(cluster=w616, "Gate Start"=w624, "Gate Stop"=w623, "Gate Step (linear only)"=w622, "Gate Compliance"=w634, "Range mode"=w599, "Range"=w598) -> (w600:T6)
        n162 = Index Array(array=w608, index #1=0 ("Index")) -> (element #1=w619:dbl, element #2=w618:dbl, element #3=w617:dbl)  [unwired: 2 in]
        n163 = call <vilib>:"compatOverwrite.vi"("overwrite (F)"=TRUE) -> ("overwrite?"=w587:T8)
        n164 = Bundle By Name(cluster=w615, "Drain Start"=w619, "Drain Stop"=w618, "Drain Step"=w617, "Drain Compliance"=w635, "Range mode"=w597, "Range"=w596) -> (w601:T7)
        n165 = call "4155C Transfer-FPP.vi"("VISA resource name in"=w603, "Gate"=w600, "Drain"=w601, "Timings"=w633, "error in (no error)"=w604, "sweep mode"=w625, "Panel Controls"=w650) -> ("VG"=w641:dbl[], "Outparams"=w595:T9, "VISA Resource Name out"=w631:refnum<visa-resource-name>, "Vprobe2"=w591:dbl[], "ID"=w590:dbl[], "IG"=w589:dbl[], "Vprobe1"=w588:dbl[], "error out"=w632:errorcluster)  [unwired: 13 in]
        n166 = Unbundle By Name(w595) -> ("V2 Step"=w594:dbl, "V2 Start"=w593:dbl, "Number of points"=w592:i32)
        n167 = Open/Create/Replace File(file path (use dialog)=w636, error in=w632, operation (0:open)=w587) -> (refnum out=w647:refnum<file>, error out=w648:errorcluster)  [unwired: 3 in, 1 out]
        n168 = call "4155C Make Big 2d array FPP.vi"("1D Var1"=w641, "1d ID"=w590, "1d Vp2"=w591, "1d IG"=w589, "1d Vp1"=w588, "VAR2 START"=w593, "Number of VAR2 steps"=w592, "VAR2 STEP"=w594, "VAR1 Name"="Vg", "Decimal places in header"=i8 1, "VAR2 Name"="Vd") -> ("Header array"=w643:string[], "Data array"=w644:dbl[][])  [unwired: 15 in]
        n169 = call "4155C Write array to file.vi"("Byte Stream File Refnum"=w647, "Header"=w643, "Data Array"=w644, "error in (no error)"=w648) -> ("dup refnum"=w645:refnum<file>, "error out"=w646:errorcluster)  [unwired: 1 in]
        n170 = Close File(refnum=w645, error in=w646) -> (error out=w630:errorcluster)  [unwired: 1 out]
      }
      frame "output" {
        # "Is off"
        # "Is on"
        # "Ig off"
        # "Ig on"
        # "Is min"
        # "Is max"
        # "Ig min"
        # "Ig max"
        # "Id min"
        # "Id max"
        # "Id off"
        # "Id on"
        n171 = Delete From Array(array=w744, index=0 ("Index")) -> (deleted portion=w742:string, array with subset deleted=w741:string[])  [unwired: 1 in]
        n172 = Bundle By Name(cluster=w656, "Emergency Stop"=w753) -> (w706:T1)
        n173 = Number To Decimal String(number=w702) -> (decimal integer string=w701:string)  [unwired: 1 in]
        n174 = case shown="\"d\", Default" w742 {
          tunnel: [w838 w839] -> w740
          frame "s" {
            w838 = u16 0 items=["Single", "Double"] ("sweep mode")
          }
          frame "d", Default {
            w839 = u16 1 items=["Single", "Double"] ("sweep mode")
          }
        }
        n175 = Fract/Exp String To Number(string=w741) -> (number=w726:dbl[])  [unwired: 3 in, 1 out]
        n176 = Concatenate Strings(w751, "-output-" ("Substring"), w701, w699, ".txt" ("Suffix (transfer)")) -> (w752:string)
        n177 = VISA Write(VISA resource name=w722, write buffer=":PAGE:CHAN:MODE SWE;" ("write buffer (\"\")"), error in (no error)=w721) -> (VISA resource name out=w719:refnum<visa-resource-name>, error out=w720:errorcluster)  [unwired: 1 out]
        n178 = String To Path(string=w752) -> (path=w750:path)
        n179 = local read "Plot output curve extrema vs time"() -> (w653:bool)
        n180 = Index Array(array=w726, index #1=0 ("Index")) -> (element #1=w739:dbl, element #2=w738:dbl, element #3=w737:dbl)  [unwired: 2 in]
        n181 = Delete From Array(array=w726, length=3 ("Length"), index=0 ("Index")) -> (array with subset deleted=w724:dbl[])  [unwired: 1 out]
        n182 = case shown="True" w653 {
          tunnel: w698 -> [w755 w758]
          tunnel: w695 -> [_ w757]
          tunnel: [w755 w756] -> w672
          frame False {
          }
          frame True {
            n183 = Build Array (concatenate)(w758, w757) -> (w756:i32[])
          }
        }
        n184 = Bundle By Name(cluster=w731, "Gate Start"=w739, "Gate Stop"=w738, "Gate Step (linear only)"=w737, "Gate Compliance"=w748, "Range mode"=w715, "Range"=w714) -> (w716:T6)
        n185 = Index Array(array=w724, index #1=0 ("Index")) -> (element #1=w734:dbl, element #2=w733:dbl, element #3=w732:dbl)  [unwired: 2 in]
        n186 = call <vilib>:"compatOverwrite.vi"("overwrite (F)"=TRUE) -> ("overwrite?"=w705:T8)
        n187 = Bundle By Name(cluster=w730, "Drain Start"=w734, "Drain Stop"=w733, "Drain Step"=w732, "Drain Compliance"=w749, "Range mode"=w713, "Range"=w712) -> (w717:T7)
        n188 = call "4155C Output.vi"("VISA resource name in"=w719, "Gate"=w716, "Drain"=w717, "Timings"=w747, "error in (no error)"=w720, "SMU4"=w707, "sweep mode"=w740, "Panel controls"=w706) -> ("VD"=w704:dbl[], "Outparams"=w711:T9, "VISA Resource Name out"=w746:refnum<visa-resource-name>, "IS"=w682:dbl[], "ID"=w683:dbl[], "IG"=w681:dbl[], "error out"=w696:errorcluster, "SMU4"=w708:dbl[])  [unwired: 12 in]
        n189 = Unbundle By Name(w711) -> ("V2 Step"=w710:dbl, "V2 Start"=w709:dbl, "Number of points"=w670:i32)
        n190 = call "4155C Split array.vi"("Number of VAR2 steps"=w670, "Y2 data in"=w683, "X data in"=w704, "Y1 data in"=w682, "Y3 data in"=w681, "error in (no error)"=w696) -> ("Array of clusters"=w697:cluster{"Y data in":dbl[], "X data in":dbl[]}[], "error out"=w658:errorcluster)  [unwired: 1 in]
        n191 = case shown="True" "Plot output curve extrema vs time" {
          tunnel: w703 -> [w767 w837]
          tunnel: w694 -> [w768 w832]
          tunnel: w685 -> [w762 w828]
          tunnel: w684 -> [w761 w827]
          tunnel: w683 -> [_ w824]
          tunnel: w682 -> [_ w822]
          tunnel: w681 -> [_ w821]
          tunnel: w680 -> [w769 w817]
          tunnel: w679 -> [w770 w816]
          tunnel: w678 -> [w765 w813]
          tunnel: w677 -> [w766 w812]
          tunnel: w676 -> [w763 w809]
          tunnel: w675 -> [w764 w808]
          tunnel: w674 -> [w759 w805]
          tunnel: w673 -> [w760 w804]
          tunnel: w672 -> [_ w797]
          tunnel: [w765 w792] -> w671
          tunnel: w670 -> [_ w791]
          tunnel: [w766 w790] -> w669
          tunnel: [w767 w789] -> w668
          tunnel: [w768 w788] -> w667
          tunnel: [w769 w787] -> w666
          tunnel: [w770 w786] -> w665
          tunnel: [w759 w785] -> w664
          tunnel: [w760 w784] -> w663
          tunnel: [w761 w783] -> w662
          tunnel: [w762 w782] -> w661
          tunnel: [w763 w781] -> w660
          tunnel: [w764 w780] -> w659
          tunnel: w658 -> [w771 w779]
          tunnel: [w771 w775] -> w657
          frame False {
          }
          frame True {
            # "Adjusts graph colors."
            # "Adjusts graph colors."
            # "Ion will be the middle element of the array. The calculation of the index is done only once, since Is, Id, and Ig have the same dimensions."
            # "abs(Ig)"
            # "abs(Is)"
            # "Y1: Is\nY2: Id\nY3: Ig"
            # "abs(Id)"
            # "Adjusts graph colors."
            # "Adjusts graph colors."
            # "Adjusts graph colors."
            n192 = Absolute Value(x=w822) -> (abs(x)=w807:dbl[])
            n193 = Absolute Value(x=w824) -> (abs(x)=w823:dbl[])
            n194 = Absolute Value(x=w821) -> (abs(x)=w810:dbl[])
            n195 = Array Size(array=w823) -> (size(s)=w831:i32)
            n196 = Divide(x=w831, y=2) -> (x/y=w774:dbl)
            n197 = Subtract(x=w774, y=1) -> (x-y=w773:dbl)
            n198 = Array Max & Min(array=w807) -> (max value=w814:dbl, min value=w815:dbl)  [unwired: 2 out]
            n199 = Array Max & Min(array=w823) -> (max value=w836:dbl, min value=w820:dbl)  [unwired: 2 out]
            n200 = Array Max & Min(array=w810) -> (max value=w819:dbl, min value=w818:dbl)  [unwired: 2 out]
            n201 = Index Array(array=w807, index=w773) -> (element=w798:dbl)
            n202 = Index Array(array=w807, index=0) -> (element=w799:dbl)
            n203 = Index Array(array=w823, index=w773) -> (element=w800:dbl)
            n204 = Index Array(array=w823, index=0) -> (element=w801:dbl)
            n205 = Index Array(array=w810, index=w773) -> (element=w803:dbl)
            n206 = Index Array(array=w810, index=0) -> (element=w802:dbl)
            n207 = local write "Ig max"(w819) -> ()
            n208 = local write "Ig min"(w818) -> ()
            n209 = local write "Is max"(w814) -> ()
            n210 = local write "Is min"(w815) -> ()
            n211 = local write "Id max"(w836) -> ()
            n212 = local write "Id min"(w820) -> ()
            n213 = Build Array (concatenate)(w813, w814) -> (w792:dbl[])
            n214 = Build Array (concatenate)(w812, w815) -> (w790:dbl[])
            n215 = local write "Is off"(w799) -> ()
            n216 = local write "Is on"(w798) -> ()
            n217 = Build Array (concatenate)(w837, w836) -> (w789:dbl[])
            n218 = Build Array (concatenate)(w832, w820) -> (w788:dbl[])
            n219 = Build Array (concatenate)(w817, w819) -> (w787:dbl[])
            n220 = Build Array (concatenate)(w816, w818) -> (w786:dbl[])
            n221 = Build Array (concatenate)(w805, w798) -> (w785:dbl[])
            n222 = Build Array (concatenate)(w804, w799) -> (w784:dbl[])
            n223 = Build Array (concatenate)(w827, w800) -> (w783:dbl[])
            n224 = Build Array (concatenate)(w828, w801) -> (w782:dbl[])
            n225 = Build Array (concatenate)(w809, w803) -> (w781:dbl[])
            n226 = Build Array (concatenate)(w808, w802) -> (w780:dbl[])
            n227 = local write "Ig off"(w802) -> ()
            n228 = local write "Ig on"(w803) -> ()
            n229 = local write "Id off"(w801) -> ()
            n230 = local write "Id on"(w800) -> ()
            n231 = control-ref of="Imax vs time"() -> (w826:refnum<vi>)
            n232 = control-ref of="Imin vs time"() -> (w825:refnum<vi>)
            n233 = control-ref of="Ion vs time"() -> (w794:refnum<vi>)
            n234 = control-ref of="Ioff vs time"() -> (w793:refnum<vi>)
            n235 = control-ref of="I vs Vg"() -> (w835:refnum<vi>)
            n236 = call "4155C Split array.vi"("Number of VAR2 steps"=w791, "Y2 data in"=w783, "X data in"=w797, "Y1 data in"=w785, "Y3 data in"=w781, "error in (no error)"=w779) -> ("Array of clusters"=w795:cluster{"Y data in":dbl[], "X data in":dbl[]}[], "error out"=w778:errorcluster)  [unwired: 1 in]
            n237 = call "4155C Split array.vi"("Number of VAR2 steps"=w791, "Y2 data in"=w782, "X data in"=w797, "Y1 data in"=w784, "Y3 data in"=w780, "error in (no error)"=w778) -> ("Array of clusters"=w796:cluster{"Y data in":dbl[], "X data in":dbl[]}[], "error out"=w777:errorcluster)  [unwired: 1 in]
            n238 = call "4155C Split array.vi"("Number of VAR2 steps"=w791, "Y2 data in"=w789, "X data in"=w797, "Y1 data in"=w792, "Y3 data in"=w787, "error in (no error)"=w777) -> ("Array of clusters"=w834:cluster{"Y data in":dbl[], "X data in":dbl[]}[], "error out"=w776:errorcluster)  [unwired: 1 in]
            n239 = call "4155C Split array.vi"("Number of VAR2 steps"=w791, "Y2 data in"=w788, "X data in"=w797, "Y1 data in"=w790, "Y3 data in"=w786, "error in (no error)"=w776) -> ("Array of clusters"=w833:cluster{"Y data in":dbl[], "X data in":dbl[]}[], "error out"=w775:errorcluster)  [unwired: 1 in]
            n240 = call "4155C Config Chart Colours.vi"("Numeric"=w791, "XY Graph 2"=w826) -> ()  [unwired: 6 in]
            n241 = call "4155C Config Chart Colours.vi"("Numeric"=w791, "XY Graph 2"=w825) -> ()  [unwired: 6 in]
            n242 = call "4155C Config Chart Colours.vi"("Numeric"=w791, "XY Graph 2"=w794) -> ()  [unwired: 6 in]
            n243 = call "4155C Config Chart Colours.vi"("Numeric"=w791, "XY Graph 2"=w793) -> ()  [unwired: 6 in]
            n244 = call "4155C Config Chart Colours.vi"("Numeric"=w791, "XY Graph 2"=w835) -> ()  [unwired: 6 in]
            n245 = local write "Imax vs time"(w834) -> ()
            n246 = local write "Imin vs time"(w833) -> ()
            n247 = local write "Ion vs time"(w795) -> ()
            n248 = local write "Ioff vs time"(w796) -> ()
          }
        }
        n249 = local write "I vs Vd"(w697) -> ()
        n250 = Open/Create/Replace File(file path (use dialog)=w750, error in=w657, operation (0:open)=w705) -> (refnum out=w692:refnum<file>, error out=w690:errorcluster)  [unwired: 3 in, 1 out]
        n251 = call "4155C Make Big 2d array.vi"("1D Var1"=w704, "1d IS"=w682, "1d ID"=w683, "1d IG"=w681, "1d SMU4"=w708, "SMU4"=w707, "VAR2 START"=w709, "Number of VAR2 steps"=w670, "VAR2 STEP"=w710, "VAR1 Name"="Vd", "Decimal places in header"=i8 1, "VAR2 Name"="Vg") -> ("Header array"=w693:string[], "Data array"=w691:dbl[][])  [unwired: 14 in]
        n252 = call "4155C Write array to file.vi"("Byte Stream File Refnum"=w692, "Header"=w693, "Data Array"=w691, "error in (no error)"=w690) -> ("dup refnum"=w689:refnum<file>, "error out"=w688:errorcluster)  [unwired: 1 in]
        n253 = Close File(refnum=w689, error in=w688) -> (error out=w745:errorcluster)  [unwired: 1 out]
      }
      frame "output-fpp" {
        n254 = Number To Decimal String(number=w854) -> (decimal integer string=w908:string)  [unwired: 1 in]
        n255 = Bundle By Name(cluster=w884, "Emergency Stop"=w911) -> (w921:T1)
        n256 = Delete From Array(array=w899, index=0 ("Index")) -> (deleted portion=w897:string, array with subset deleted=w896:string[])  [unwired: 1 in]
        n257 = VISA Write(VISA resource name=w875, write buffer=":PAGE:CHAN:MODE SWE;" ("write buffer (\"\")"), error in (no error)=w872) -> (VISA resource name out=w874:refnum<visa-resource-name>, error out=w873:errorcluster)  [unwired: 1 out]
        n258 = Concatenate Strings(w907, "-outputfpp-" ("Substring"), w908, w853, ".txt" ("Substring")) -> (w910:string)
        n259 = case shown="\"d\", Default" w897 {
          tunnel: [w922 w923] -> w895
          frame "s" {
            w922 = u16 0 items=["Single", "Double"] ("sweep mode")
          }
          frame "d", Default {
            w923 = u16 1 items=["Single", "Double"] ("sweep mode")
          }
        }
        n260 = Fract/Exp String To Number(string=w896) -> (number=w878:dbl[])  [unwired: 3 in, 1 out]
        n261 = String To Path(string=w910) -> (path=w906:path)
        n262 = Index Array(array=w878, index #1=0 ("Index")) -> (element #1=w894:dbl, element #2=w893:dbl, element #3=w892:dbl)  [unwired: 2 in]
        n263 = Delete From Array(array=w878, length=3 ("Length"), index=0 ("Index")) -> (array with subset deleted=w877:dbl[])  [unwired: 1 out]
        n264 = Bundle By Name(cluster=w886, "Gate Start"=w894, "Gate Stop"=w893, "Gate Step (linear only)"=w892, "Gate Compliance"=w904, "Range mode"=w870, "Range"=w869) -> (w920:T6)
        n265 = Index Array(array=w877, index #1=0 ("Index")) -> (element #1=w889:dbl, element #2=w888:dbl, element #3=w887:dbl)  [unwired: 2 in]
        n266 = call <vilib>:"compatOverwrite.vi"("overwrite (F)"=TRUE) -> ("overwrite?"=w858:T8)
        n267 = Bundle By Name(cluster=w885, "Drain Start"=w889, "Drain Stop"=w888, "Drain Step"=w887, "Drain Compliance"=w905, "Range mode"=w868, "Range"=w871) -> (w919:T7)
        n268 = call "4155C Output-FPP.vi"("VISA resource name in"=w874, "Gate"=w920, "Drain"=w919, "Timings"=w903, "error in (no error)"=w873, "sweep mode"=w895, "Panel controls"=w921) -> ("VD"=w863:dbl[], "Outparams"=w866:T9, "VISA Resource Name out"=w901:refnum<visa-resource-name>, "Vprobe2"=w862:dbl[], "ID"=w861:dbl[], "IG"=w860:dbl[], "Vprobe1"=w859:dbl[], "error out"=w902:errorcluster)  [unwired: 13 in]
        n269 = Unbundle By Name(w866) -> ("V2 Step"=w867:dbl, "V2 Start"=w865:dbl, "Number of points"=w864:i32)
        n270 = Open/Create/Replace File(file path (use dialog)=w906, error in=w902, operation (0:open)=w858) -> (refnum out=w916:refnum<file>, error out=w917:errorcluster)  [unwired: 3 in, 1 out]
        n271 = call "4155C Make Big 2d array FPP.vi"("1D Var1"=w863, "1d ID"=w861, "1d Vp2"=w862, "1d IG"=w860, "1d Vp1"=w859, "VAR2 START"=w865, "Number of VAR2 steps"=w864, "VAR2 STEP"=w867, "VAR1 Name"="Vd", "Decimal places in header"=i8 1, "VAR2 Name"="Vg") -> ("Header array"=w912:string[], "Data array"=w913:dbl[][])  [unwired: 15 in]
        n272 = call "4155C Write array to file.vi"("Byte Stream File Refnum"=w916, "Header"=w912, "Data Array"=w913, "error in (no error)"=w917) -> ("dup refnum"=w914:refnum<file>, "error out"=w915:errorcluster)  [unwired: 1 in]
        n273 = Close File(refnum=w914, error in=w915) -> (error out=w900:errorcluster)  [unwired: 1 out]
      }
      frame "itime" {
        n274 = Delete From Array(array=w926, index=1) -> (deleted portion=w925:string)  [unwired: 1 in, 1 out]
        n275 = Delete From Array(array=w926, index=0 ("Index")) -> (deleted portion=w954:string)  [unwired: 1 in, 1 out]
        n276 = Fract/Exp String To Number(string=w925) -> (number=w924:dbl)  [unwired: 3 in, 1 out]
        n277 = case shown="\"l\"" w954 {
          tunnel: w953 -> [w959 w961 w965]
          tunnel: [w958 w960 w964] -> w946
          tunnel: w924 -> [w956 _ w963]
          frame "s" {
            w957 = u32 0 items=["short  ", "medium  ", "long  "] ("integration time 2")
            n278 = Bundle By Name(cluster=w959, "integration time"=w957, "Short/Long integration time"=w956) -> (w958:T4)
          }
          frame "m", Default {
            w962 = u32 1 items=["short  ", "medium  ", "long  "] ("integration time 2")
            n279 = Bundle By Name(cluster=w961, "integration time"=w962) -> (w960:T4)
          }
          frame "l" {
            w966 = u32 2 items=["short  ", "medium  ", "long  "] ("integration time 2")
            n280 = Bundle By Name(cluster=w965, "integration time"=w966, "Short/Long integration time"=w963) -> (w964:T4)
          }
        }
      }
      frame "pulsed" {
        n281 = Delete From Array(array=w994, index=0 ("Index")) -> (deleted portion=w995:string, array with subset deleted=w982:string[])  [unwired: 1 in]
        n282 = case shown="\"on\", Default" w995 {
          tunnel: w993 -> [w1005 w1008]
          tunnel: [w1004 w1007] -> w986
          tunnel: w982 -> [w1002 _]
          frame "on", Default {
            w1003 = u16 1 items=["Continuous", "Pulsed"] ("sweep method")
            n283 = Fract/Exp String To Number(string=w1002) -> (number=w1000:dbl[])  [unwired: 3 in, 1 out]
            n284 = Index Array(array=w1000, index #1=0 ("Index")) -> (element #1=w999:dbl, element #2=w998:dbl, element #3=w997:dbl)  [unwired: 2 in]
            n285 = Bundle By Name(cluster=w1005, "sweep method"=w1003, "Pulse period"=w999, "Base voltage"=w998, "Pulse width"=w997) -> (w1004:T4)
          }
          frame "off" {
            w1006 = u16 0 items=["Continuous", "Pulsed"] ("sweep method")
            n286 = Bundle By Name(cluster=w1008, "sweep method"=w1006) -> (w1007:T4)
          }
        }
      }
      frame "gaterangemode" {
        n287 = Delete From Array(array=w1034, index=0 ("Index")) -> (deleted portion=w1035:string)  [unwired: 1 in, 1 out]
        n288 = case shown="\"f\"" w1035 {
          tunnel: [w1037 w1038 w1039] -> w1024
          frame "a", Default {
            w1037 = u16 0 items=["Auto", "Limited", "Fixed"] ("Gate Range\nmode 2")
          }
          frame "f" {
            w1038 = u16 2 items=["Auto", "Limited", "Fixed"] ("Gate Range\nmode 2")
          }
          frame "l" {
            w1039 = u16 1 items=["Auto", "Limited", "Fixed"] ("Gate Range\nmode 2")
          }
        }
      }
      frame "gaterange" {
        (unwired) u8 11 items=["10fA  ", "100fA  ", "1nA  ", "10nA", "100nA", "1uA", "10uA", "100uA", "1mA", "10mA", "100mA", "1A"] ("Gate Range 2")
        n289 = Delete From Array(array=w1072, index=0 ("Index")) -> (deleted portion=w1062:string)  [unwired: 1 in, 1 out]
        n290 = Scan Value(string=w1062, format string="") -> (value=w1060:dbl)  [unwired: 1 in, 1 out]
        n291 = Logarithm Base 10(1:w1060) -> (0:w1059:dbl)
        n292 = Round To Nearest(number=w1059) -> (nearest integer value=w1058:dbl)
        n293 = Add(x=w1058, y=11.0) -> (x+y=w1056:dbl)
        n294 = To Unsigned Byte Integer(number=w1056) -> (unsigned 8bit integer=w1055:u8)
      }
      frame "drainrange" {
        (unwired) u8 11 items=["10fA  ", "100fA  ", "1nA  ", "10nA", "100nA", "1uA", "10uA", "100uA", "1mA", "10mA", "100mA", "1A"] ("Gate Range 2")
        n295 = Delete From Array(array=w1106, index=0 ("Index")) -> (deleted portion=w1097:string)  [unwired: 1 in, 1 out]
        n296 = Scan Value(string=w1097, format string="") -> (value=w1095:dbl)  [unwired: 1 in, 1 out]
        n297 = Logarithm Base 10(1:w1095) -> (0:w1094:dbl)
        n298 = Round To Nearest(number=w1094) -> (nearest integer value=w1093:dbl)
        n299 = Add(x=w1093, y=11.0) -> (x+y=w1091:dbl)
        n300 = To Unsigned Byte Integer(number=w1091) -> (unsigned 8bit integer=w1090:u8)
      }
      frame "drainrangemode" {
        n301 = Delete From Array(array=w1133, index=0 ("Index")) -> (deleted portion=w1134:string)  [unwired: 1 in, 1 out]
        n302 = case shown="\"f\"" w1134 {
          tunnel: [w1136 w1137 w1138] -> w1123
          frame "a", Default {
            w1136 = u16 0 items=["Auto", "Limited", "Fixed"] ("Gate Range\nmode 2")
          }
          frame "f" {
            w1137 = u16 2 items=["Auto", "Limited", "Fixed"] ("Gate Range\nmode 2")
          }
          frame "l" {
            w1138 = u16 1 items=["Auto", "Limited", "Fixed"] ("Gate Range\nmode 2")
          }
        }
      }
      frame "Error", Default {
      }
      frame "logfile" {
        n303 = Number To Decimal String(number=w1179) -> (decimal integer string=w1214:string)  [unwired: 1 in]
        n304 = Concatenate Strings(w1213, "logfile" ("Substring"), w1214, w1177, ".txt" ("Substring")) -> (w1211:string)
        n305 = String To Path(string=w1211) -> (path=w1184:path)
        n306 = Unbundle(w1210) -> ("integration time"=w1209:u32, "Short/Long integration time"=w1208:dbl, "hold time (sec)"=w1207:dbl, "delay time (sec)"=w1206:dbl, "Step Time (0 disables)"=w1205:dbl, "sweep method"=w1204:u16, "Pulse period"=w1203:dbl, "Base voltage"=w1202:dbl, "Pulse width"=w1201:dbl)
        n307 = Build Array(w1209, w1208, w1207, w1206, w1205, w1204, w1203, w1202, w1201, w1195, w1196, w1197, w1198, w1199, w1200) -> (w1188:dbl[])
        n308 = Insert Into Array(array=dbl[][] [] ("Input Array"), new element=w1188) -> (w1187:dbl[][])  [unwired: 2 in]
        n309 = call <vilib>:"compatOverwrite.vi"("overwrite (F)"=TRUE) -> ("overwrite?"=w1182:T8)
        n310 = Open/Create/Replace File(file path (use dialog)=w1184, error in=w1186, operation (0:open)=w1182) -> (refnum out=w1192:refnum<file>, error out=w1191:errorcluster)  [unwired: 3 in, 1 out]
        n311 = call "4155C Write array to file.vi"("Byte Stream File Refnum"=w1192, "Header"=string[] ["Int Time", "Short/Long Itime", "Hold time", "Delay time", "Step time", "Sweep method", "Pulse period", "Base Voltage", "Pulse width", "Drain compliance", "Gate compliance", "Gate range mode", "Gate range", "S/D range mode", "S/D range"], "Data Array"=w1187, "error in (no error)"=w1191) -> ("dup refnum"=w1194:refnum<file>, "error out"=w1193:errorcluster)  [unwired: 1 in]
        n312 = Close File(refnum=w1194, error in=w1193) -> (error out=w1185:errorcluster)  [unwired: 1 out]
      }
      frame "sample" {
        n313 = Number To Decimal String(number=w1231) -> (decimal integer string=w1279:string)  [unwired: 1 in]
        n314 = Fract/Exp String To Number(string=w1276) -> (number=w1237:dbl[])  [unwired: 3 in, 1 out]
        n315 = Concatenate Strings(w1254, "-sample-" ("Substring"), w1279, w1229, ".txt" ("Substring")) -> (w1277:string)
        n316 = Index Array(array=w1237, index=0 ("Index")) -> (element=w1274:dbl)
        n317 = String To Path(string=w1277) -> (path=w1258:path)
        n318 = Index Array(array=w1237, index=2 ("Index")) -> (element=w1270:dbl)
        n319 = Index Array(array=w1237, index=3 ("Index")) -> (element=w1239:dbl)
        n320 = Index Array(array=w1237, index=4 ("Index")) -> (element=w1236:dbl)
        n321 = call "4155C Config Sampling Measurements.vi"("Sampling interval"=w1236, "Sample time"=w1239, "Display on/off"=TRUE, "Timings"=w1245, "Num Points"=w1270, "error in (no error)"=w1281, "Drain Compliance"=w1280, "Gate Compliance"=w1255, "VISA session"=w1282) -> ("error out"=w1283:errorcluster, "dup VISA resource name"=w1284:refnum<visa-resource-name>)  [unwired: 1 in]
        n322 = Index Array(array=w1237, index=1 ("Index")) -> (element=w1271:dbl)
        n323 = call "4155C Take Sample.vi"("Emergency Stop"=w1251, "error in (no error)"=w1283, "Vd"=w1271, "Vg"=w1274, "VISA resource name in"=w1284) -> ("error out"=w1249:errorcluster, "Id"=w1286:dbl[], "Ig"=w1260:dbl[], "VISA Resource Name out"=w1247:refnum<visa-resource-name>, "Is"=w1285:dbl[], "Time"=w1264:dbl[])  [unwired: 1 in]
        n324 = Insert Into Array(array=dbl[][] [] ("Input Array"), new element=w1264) -> (w1263:dbl[][])  [unwired: 2 in]
        n325 = Insert Into Array(array=w1263, new element=w1260) -> (w1262:dbl[][])  [unwired: 2 in]
        n326 = Insert Into Array(array=w1262, new element=w1286) -> (w1261:dbl[][])  [unwired: 2 in]
        n327 = VISA Write(VISA resource name=w1247, write buffer=":DISP ON" ("write buffer (\"\")"), error in (no error)=w1249) -> (VISA resource name out=w1246:refnum<visa-resource-name>, error out=w1248:errorcluster)  [unwired: 1 out]
        n328 = Insert Into Array(array=w1261, new element=w1285) -> (w1253:dbl[][])  [unwired: 2 in]
        n329 = Transpose 2D Array(2D array=w1253) -> (transposed array=w1252:dbl[][])
        n330 = call <vilib>:"compatOverwrite.vi"("overwrite (F)"=TRUE) -> ("overwrite?"=w1234:T8)
        n331 = Open/Create/Replace File(file path (use dialog)=w1258, error in=w1248, operation (0:open)=w1234) -> (refnum out=w1267:refnum<file>, error out=w1266:errorcluster)  [unwired: 3 in, 1 out]
        n332 = call "4155C Write array to file.vi"("Byte Stream File Refnum"=w1267, "Header"=string[] ["Time /s", "Ig /A", "Id /A", "Is /A"], "Data Array"=w1252, "error in (no error)"=w1266) -> ("dup refnum"=w1269:refnum<file>, "error out"=w1268:errorcluster)  [unwired: 1 in]
        n333 = Close File(refnum=w1269, error in=w1268) -> (error out=w1256:errorcluster)  [unwired: 1 out]
      }
      frame "samplei" {
        n334 = Number To Decimal String(number=w1302) -> (decimal integer string=w1353:string)  [unwired: 1 in]
        n335 = Concatenate Strings(w1332, "-samplei-" ("Substring"), w1353, w1301, ".txt" ("Substring")) -> (w1351:string)
        n336 = Fract/Exp String To Number(string=w1350) -> (number=w1317:dbl[])  [unwired: 3 in, 1 out]
        n337 = String To Path(string=w1351) -> (path=w1335:path)
        n338 = Index Array(array=w1317, index=4 ("Index")) -> (element=w1311:dbl)
        n339 = Index Array(array=w1317, index=3 ("Index")) -> (element=w1312:dbl)
        n340 = Index Array(array=w1317, index=1 ("Index")) -> (element=w1314:dbl)
        n341 = Index Array(array=w1317, index=0 ("Index")) -> (element=w1315:dbl)
        n342 = Index Array(array=w1317, index=2 ("Index")) -> (element=w1313:dbl)
        n343 = call "4155C Config SamplingI Measurements.vi"("Sample time"=w1313, "Display on/off"=TRUE, "Timings"=w1324, "Num Points"=w1314, "error in (no error)"=w1355, "Sampling interval"=w1312, "VISA session"=w1356) -> ("error out"=w1357:errorcluster, "dup VISA resource name"=w1358:refnum<visa-resource-name>)  [unwired: 3 in]
        n344 = call "4155C Take SampleI.vi"("Emergency Stop"=w1329, "error in (no error)"=w1357, "Idg 2"=w1315, "Vdg compliance 2"=w1311, "VISA resource name in"=w1358) -> ("error out"=w1327:errorcluster, "Idg"=w1360:dbl[], "Vdg"=w1337:dbl[], "VISA Resource Name out"=w1325:refnum<visa-resource-name>, "Is"=w1359:dbl[], "Time"=w1341:dbl[])  [unwired: 1 in]
        n345 = Insert Into Array(array=dbl[][] [] ("Input Array"), new element=w1341) -> (w1340:dbl[][])  [unwired: 2 in]
        n346 = Insert Into Array(array=w1340, new element=w1337) -> (w1339:dbl[][])  [unwired: 2 in]
        n347 = Insert Into Array(array=w1339, new element=w1360) -> (w1338:dbl[][])  [unwired: 2 in]
        n348 = VISA Write(VISA resource name=w1325, write buffer=":DISP ON" ("write buffer (\"\")"), error in (no error)=w1327) -> (VISA resource name out=w1310:refnum<visa-resource-name>, error out=w1326:errorcluster)  [unwired: 1 out]
        n349 = Insert Into Array(array=w1338, new element=w1359) -> (w1331:dbl[][])  [unwired: 2 in]
        n350 = call <vilib>:"compatOverwrite.vi"("overwrite (F)"=TRUE) -> ("overwrite?"=w1305:T8)
        n351 = Open/Create/Replace File(file path (use dialog)=w1335, error in=w1326, operation (0:open)=w1305) -> (refnum out=w1344:refnum<file>, error out=w1343:errorcluster)  [unwired: 3 in, 1 out]
        n352 = Transpose 2D Array(2D array=w1331) -> (transposed array=w1330:dbl[][])
        n353 = call "4155C Write array to file.vi"("Byte Stream File Refnum"=w1344, "Header"=string[] ["Time /s", "Vdg /V", "Idg /A", "Is /A"], "Data Array"=w1330, "error in (no error)"=w1343) -> ("dup refnum"=w1346:refnum<file>, "error out"=w1345:errorcluster)  [unwired: 1 in]
        n354 = Close File(refnum=w1346, error in=w1345) -> (error out=w1308:errorcluster)  [unwired: 1 out]
        n355 = VISA Write(VISA resource name=w1310, write buffer=";:PAGE:SCON:STAN OFF;:PAGE:CHAN:VSU2:DIS;" ("write buffer (\"\")"), error in (no error)=w1308) -> (VISA resource name out=w1306:refnum<visa-resource-name>, error out=w1307:errorcluster)  [unwired: 1 out]
      }
      frame "#" {
        n356 = VISA Write(VISA resource name=w1380, write buffer=":DISP ON" ("write buffer (\"\")"), error in (no error)=w1379) -> (VISA resource name out=w1378:refnum<visa-resource-name>, error out=w1377:errorcluster)  [unwired: 1 out]
      }
      frame "stressV" {
        n357 = Number To Decimal String(number=w1403) -> (decimal integer string=w1444:string)  [unwired: 1 in]
        n358 = Concatenate Strings(w1428, "-stressV-" ("Substring"), w1444, w1402, ".txt" ("Substring")) -> (w1442:string)
        n359 = Fract/Exp String To Number(string=w1441) -> (number=w1414:dbl[])  [unwired: 3 in, 1 out]
        n360 = String To Path(string=w1442) -> (path=w1432:path)
        n361 = Index Array(array=w1414, index=3 ("Index")) -> (element=w1411:dbl)
        n362 = Index Array(array=w1414, index=1 ("Index")) -> (element=w1409:dbl)
        n363 = Index Array(array=w1414, index=0 ("Index")) -> (element=w1408:dbl)
        n364 = Index Array(array=w1414, index=4 ("Index")) -> (element=w1413:dbl)
        n365 = Index Array(array=w1414, index=2 ("Index")) -> (element=w1410:dbl)
        n366 = call "4155C Config V Stress.vi"("VISA session"=w1447, "ID compliance"=w1411, "VD"=w1409, "VG"=w1408, "IG compliance"=w1410, "error in (no error)"=w1446, "Display on/off"=TRUE) -> ("dup VISA resource name"=w1449:refnum<visa-resource-name>, "error out"=w1448:errorcluster)
        n367 = call "4155C Apply Stress.vi"("error in (no error)"=w1448, "Duration"=w1413, "Emergency Stop"=w1427, "VISA resource name in"=w1449) -> ("error out"=w1425:errorcluster, "VISA Resource Name out"=w1423:refnum<visa-resource-name>)
        n368 = VISA Write(VISA resource name=w1423, write buffer=":DISP ON" ("write buffer (\"\")"), error in (no error)=w1425) -> (VISA resource name out=w1422:refnum<visa-resource-name>, error out=w1424:errorcluster)  [unwired: 1 out]
        n369 = call <vilib>:"compatOverwrite.vi"("overwrite (F)"=TRUE) -> ("overwrite?"=w1407:T8)
        n370 = Open/Create/Replace File(file path (use dialog)=w1432, error in=w1424, operation (0:open)=w1407) -> (refnum out=w1435:refnum<file>, error out=w1434:errorcluster)  [unwired: 3 in, 1 out]
        n371 = call "4155C Write array to file.vi"("Byte Stream File Refnum"=w1435, "Header"=string[] ["V stress completed successfully", ""], "error in (no error)"=w1434) -> ("dup refnum"=w1437:refnum<file>, "error out"=w1436:errorcluster)  [unwired: 2 in]
        n372 = Close File(refnum=w1437, error in=w1436) -> (error out=w1430:errorcluster)  [unwired: 1 out]
      }
      frame "stressI" {
        n373 = Number To Decimal String(number=w1464) -> (decimal integer string=w1501:string)  [unwired: 1 in]
        n374 = Concatenate Strings(w1485, "-stressI-" ("Substring"), w1501, w1463, ".txt" ("Substring")) -> (w1499:string)
        n375 = Fract/Exp String To Number(string=w1498) -> (number=w1473:dbl[])  [unwired: 3 in, 1 out]
        n376 = Index Array(array=w1473, index=1 ("Index")) -> (element=w1469:dbl)
        n377 = Index Array(array=w1473, index=0 ("Index")) -> (element=w1470:dbl)
        n378 = call "4155C Config I Stress.vi"("VISA session"=w1504, "IDG"=w1470, "VDG compliance"=w1469, "error in (no error)"=w1503, "Display on/off"=TRUE) -> ("dup VISA resource name"=w1506:refnum<visa-resource-name>, "error out"=w1505:errorcluster)
        n379 = Index Array(array=w1473, index=2 ("Index")) -> (element=w1471:dbl)
        n380 = String To Path(string=w1499) -> (path=w1489:path)
        n381 = call "4155C Apply Stress.vi"("error in (no error)"=w1505, "Duration"=w1471, "Emergency Stop"=w1484, "VISA resource name in"=w1506) -> ("error out"=w1482:errorcluster, "VISA Resource Name out"=w1480:refnum<visa-resource-name>)
        n382 = VISA Write(VISA resource name=w1480, write buffer=":DISP ON" ("write buffer (\"\")"), error in (no error)=w1482) -> (VISA resource name out=w1479:refnum<visa-resource-name>, error out=w1481:errorcluster)  [unwired: 1 out]
        n383 = call <vilib>:"compatOverwrite.vi"("overwrite (F)"=TRUE) -> ("overwrite?"=w1468:T8)
        n384 = Open/Create/Replace File(file path (use dialog)=w1489, error in=w1481, operation (0:open)=w1468) -> (refnum out=w1492:refnum<file>, error out=w1491:errorcluster)  [unwired: 3 in, 1 out]
        n385 = call "4155C Write array to file.vi"("Byte Stream File Refnum"=w1492, "Header"=string[] ["I stress completed successfully", ""], "error in (no error)"=w1491) -> ("dup refnum"=w1494:refnum<file>, "error out"=w1493:errorcluster)  [unwired: 2 in]
        n386 = Close File(refnum=w1494, error in=w1493) -> (error out=w1487:errorcluster)  [unwired: 1 out]
      }
      frame "vsu2pulse" {
        n387 = Number To Decimal String(number=w1521) -> (decimal integer string=w1556:string)  [unwired: 1 in]
        n388 = Concatenate Strings(w1541, "-vsu2-" ("Substring"), w1556, w1520, ".txt" ("Substring")) -> (w1554:string)
        n389 = Fract/Exp String To Number(string=w1553) -> (number=w1529:dbl[])  [unwired: 3 in, 1 out]
        n390 = String To Path(string=w1554) -> (path=w1545:path)
        n391 = Index Array(array=w1529, index=1 ("Index")) -> (element=w1528:dbl)
        n392 = Index Array(array=w1529, index=0 ("Index")) -> (element=w1526:dbl)
        n393 = call "4155C Config VSU2 Stress.vi"("error in (no error)"=w1558, "VSU2"=w1526, "Display on/off"=TRUE, "VISA session"=w1559) -> ("error out"=w1560:errorcluster, "dup VISA resource name"=w1561:refnum<visa-resource-name>)
        n394 = call "4155C Apply Stress.vi"("error in (no error)"=w1560, "Duration"=w1528, "Emergency Stop"=w1540, "VISA resource name in"=w1561) -> ("error out"=w1538:errorcluster, "VISA Resource Name out"=w1536:refnum<visa-resource-name>)
        n395 = VISA Write(VISA resource name=w1536, write buffer=":DISP ON" ("write buffer (\"\")"), error in (no error)=w1538) -> (VISA resource name out=w1535:refnum<visa-resource-name>, error out=w1537:errorcluster)  [unwired: 1 out]
        n396 = call <vilib>:"compatOverwrite.vi"("overwrite (F)"=TRUE) -> ("overwrite?"=w1525:T8)
        n397 = Open/Create/Replace File(file path (use dialog)=w1545, error in=w1537, operation (0:open)=w1525) -> (refnum out=w1548:refnum<file>, error out=w1547:errorcluster)  [unwired: 3 in, 1 out]
        n398 = call "4155C Write array to file.vi"("Byte Stream File Refnum"=w1548, "Header"=string[] ["VSU2 pulse completed successfully", ""], "error in (no error)"=w1547) -> ("dup refnum"=w1550:refnum<file>, "error out"=w1549:errorcluster)  [unwired: 2 in]
        n399 = Close File(refnum=w1550, error in=w1549) -> (error out=w1543:errorcluster)  [unwired: 1 out]
      }
      frame "sample-fpp" {
        w1587 = string[] ["Time /s", "Id VgVd /A", "Ig VgVd /A", "Vp1 VgVd /V", "Vp2 VgVd /V"] ("Header")
        w1591 = "%d" ("format string")
        n400 = Number To Decimal String(number=w1576) -> (decimal integer string=w1639:string)  [unwired: 1 in]
        n401 = Fract/Exp String To Number(string=w1636) -> (number=w1624:dbl[])  [unwired: 3 in, 1 out]
        n402 = Concatenate Strings(w1630, "-samplefpp-" ("Substring"), w1639, w1575, ".txt" ("Substring")) -> (w1637:string)
        n403 = String To Path(string=w1637) -> (path=w1599:path)
        n404 = Index Array(array=w1624, index=0 ("Index")) -> (element=w1585:dbl)
        n405 = Index Array(array=w1624, index=1 ("Index")) -> (element=w1584:dbl)
        n406 = Index Array(array=w1624, index=2 ("Index")) -> (element=w1632:dbl)
        n407 = Index Array(array=w1624, index=3 ("Index")) -> (element=w1622:dbl)
        n408 = call "4155C Config Sampling Measurements FPP.vi"("VISA session"=w1642, "Num Points"=w1632, "Vg"=w1585, "Display on/off"=TRUE, "Gate Compliance"=w1631, "Drain Compliance"=w1640, "Standby"="Standby", "error in (no error)"=w1641, "Timings"=w1629, "Vd"=w1584, "Sample time"=w1622) -> ("dup VISA resource name"=w1601:refnum<visa-resource-name>, "error out"=w1600:errorcluster)  [unwired: 3 in]
        n409 = Number To Decimal String(number=w1585) -> (decimal integer string=w1611:string)  [unwired: 1 in]
        n410 = call "4155C Take Sample FPP.vi"("VISA resource name in"=w1601, "error in (no error)"=w1600, "Emergency Stop"=w1602) -> ("Time"=w1606:dbl[], "Vp1"=w1616:dbl[], "VISA Resource Name out"=w1582:refnum<visa-resource-name>, "Ig"=w1604:dbl[], "Id"=w1605:dbl[], "Vp2"=w1614:dbl[], "error out"=w1603:errorcluster)  [unwired: 10 in]
        n411 = Insert Into Array(array=dbl[][] [] ("Input Array"), new element=w1606) -> (w1620:dbl[][])  [unwired: 2 in]
        n412 = Number To Decimal String(number=w1584) -> (decimal integer string=w1609:string)  [unwired: 1 in]
        n413 = Insert Into Array(array=w1620, new element=w1605) -> (w1619:dbl[][])  [unwired: 2 in]
        n414 = Concatenate Strings("(Vg = " ("Substring"), w1611, "V, Vd = " ("Substring"), w1609, "V)" ("Substring")) -> (w1607:string)
        n415 = Insert Into Array(array=w1619, new element=w1604) -> (w1618:dbl[][])  [unwired: 2 in]
        n416 = Insert Into Array(array=w1618, new element=w1616) -> (w1615:dbl[][])  [unwired: 2 in]
        n417 = Insert Into Array(array=w1615, new element=w1614) -> (w1583:dbl[][])  [unwired: 2 in]
        n418 = Transpose 2D Array(2D array=w1583) -> (transposed array=w1613:dbl[][])
        n419 = call <vilib>:"compatOverwrite.vi"("overwrite (F)"=TRUE) -> ("overwrite?"=w1580:T8)
        n420 = Open/Create/Replace File(file path (use dialog)=w1599, error in=w1603, operation (0:open)=w1580) -> (refnum out=w1596:refnum<file>, error out=w1597:errorcluster)  [unwired: 3 in, 1 out]
        n421 = Array To Spreadsheet String(array=w1587, 3:w1591) -> (spreadsheet string=w1593:string)  [unwired: 1 in]
        n422 = Search and Replace String(replace all?=TRUE ("replace all? (F)"), input string=w1593, search string="VgVd", replace string=w1607) -> (result string=w1589:string)  [unwired: 4 in, 3 out]
        n423 = Spreadsheet String To Array(format string=w1591, spreadsheet string=w1589, array type (2D Dbl)=w1587) -> (array=w1588:string[])  [unwired: 1 in]
        n424 = call "4155C Write array to file.vi"("Byte Stream File Refnum"=w1596, "Header"=w1588, "Data Array"=w1613, "error in (no error)"=w1597) -> ("dup refnum"=w1594:refnum<file>, "error out"=w1595:errorcluster)  [unwired: 1 in]
        n425 = Close File(refnum=w1594, error in=w1595) -> (error out=w1581:errorcluster)  [unwired: 1 out]
      }
      frame "resample-fpp" {
        w1670 = string[] ["Time /s", "Id VgVd /A", "Ig VgVd /A", "Vp1 VgVd /V", "Vp2 VgVd /V"] ("Header")
        w1674 = "%d" ("format string")
        n426 = Number To Decimal String(number=w1656) -> (decimal integer string=w1714:string)  [unwired: 1 in]
        n427 = Fract/Exp String To Number(string=w1711) -> (number=w1663:dbl[])  [unwired: 3 in, 1 out]
        n428 = Concatenate Strings(w1707, "-resamplefpp-" ("Substring"), w1714, w1657, ".txt" ("Substring")) -> (w1712:string)
        n429 = String To Path(string=w1712) -> (path=w1682:path)
        n430 = Index Array(array=w1663, index=0 ("Index")) -> (element=w1669:dbl)
        n431 = Index Array(array=w1663, index=1 ("Index")) -> (element=w1668:dbl)
        n432 = Number To Decimal String(number=w1669) -> (decimal integer string=w1692:string)  [unwired: 1 in]
        n433 = call "4155C Take Sample FPP.vi"("VISA resource name in"=w1665, "error in (no error)"=w1664, "Emergency Stop"=w1683) -> ("Time"=w1687:dbl[], "Vp1"=w1697:dbl[], "VISA Resource Name out"=w1667:refnum<visa-resource-name>, "Ig"=w1685:dbl[], "Id"=w1686:dbl[], "Vp2"=w1695:dbl[], "error out"=w1684:errorcluster)  [unwired: 10 in]
        n434 = Insert Into Array(array=dbl[][] [] ("Input Array"), new element=w1687) -> (w1701:dbl[][])  [unwired: 2 in]
        n435 = Number To Decimal String(number=w1668) -> (decimal integer string=w1690:string)  [unwired: 1 in]
        n436 = Insert Into Array(array=w1701, new element=w1686) -> (w1700:dbl[][])  [unwired: 2 in]
        n437 = Concatenate Strings("(Vg = " ("Substring"), w1692, "V, Vd = " ("Substring"), w1690, "V)" ("Substring")) -> (w1688:string)
        n438 = Insert Into Array(array=w1700, new element=w1685) -> (w1699:dbl[][])  [unwired: 2 in]
        n439 = Insert Into Array(array=w1699, new element=w1697) -> (w1696:dbl[][])  [unwired: 2 in]
        n440 = Insert Into Array(array=w1696, new element=w1695) -> (w1662:dbl[][])  [unwired: 2 in]
        n441 = call <vilib>:"compatOverwrite.vi"("overwrite (F)"=TRUE) -> ("overwrite?"=w1661:T8)
        n442 = Open/Create/Replace File(file path (use dialog)=w1682, error in=w1684, operation (0:open)=w1661) -> (refnum out=w1679:refnum<file>, error out=w1680:errorcluster)  [unwired: 3 in, 1 out]
        n443 = Array To Spreadsheet String(array=w1670, 3:w1674) -> (spreadsheet string=w1676:string)  [unwired: 1 in]
        n444 = Transpose 2D Array(2D array=w1662) -> (transposed array=w1694:dbl[][])
        n445 = Search and Replace String(replace all?=TRUE ("replace all? (F)"), input string=w1676, search string="VgVd", replace string=w1688) -> (result string=w1672:string)  [unwired: 4 in, 3 out]
        n446 = Spreadsheet String To Array(format string=w1674, spreadsheet string=w1672, array type (2D Dbl)=w1670) -> (array=w1671:string[])  [unwired: 1 in]
        n447 = call "4155C Write array to file.vi"("Byte Stream File Refnum"=w1679, "Header"=w1671, "Data Array"=w1694, "error in (no error)"=w1680) -> ("dup refnum"=w1677:refnum<file>, "error out"=w1678:errorcluster)  [unwired: 1 in]
        n448 = Close File(refnum=w1677, error in=w1678) -> (error out=w1666:errorcluster)  [unwired: 1 out]
      }
      frame "serial" {
        n449 = local read "Termination char\n(0xA = '\\n' = LF)\n(0xD = '\\r' = CR)"() -> (w1736:u8)
        n450 = local read "Enable Termination\nChar (T)"() -> (w1737:bool)
        n451 = Index Array(array=w1744, index=0 ("Index")) -> (element=w1743:string)
        n452 = local read "parity"() -> (w1727:u16)
        n453 = local read "Delay before read (ms)"() -> (w1738:u32)
        n454 = local read "byte count"() -> (w1735:u32)
        n455 = local read "Timeout (ms)"() -> (w1734:u32)
        n456 = local read "VISA resource name"() -> (w1731:refnum<visa-resource-name>)
        n457 = local read "baud rate"() -> (w1730:u32)
        n458 = local read "Serial End Mode for Reads"() -> (w1729:u16)
        n459 = local read "data bits"() -> (w1728:u16)
        n460 = local read "stop bits"() -> (w1733:u16)
        n461 = local read "flow control"() -> (w1732:u16)
        n462 = call "Serial write and read v0.5.vi"("Delay before read (ms)"=w1738, "Termination char\n(0xA = '\\n' = LF)\n(0xD = '\\r' = CR)"=w1736, "Enable Termination\nChar (T)"=w1737, "parity"=w1727, "stop bits"=w1733, "string to write"=w1743, "flow control"=w1732, "byte count"=w1735, "Serial Settings:Serial End Mode for Reads"=w1729, "Timeout (ms)"=w1734, "error in (no error)"=w1749, "VISA resource name"=w1731, "baud rate"=w1730, "data bits"=w1728) -> ("Serial port output"=w1739:string, "error out"=w1748:errorcluster)
        n463 = Build Array (concatenate)(w1739, w1740) -> (w1741:string[])
      }
    }
    n464 = local read "Time Units"() -> (w64:u16)
    n465 = case shown="0" w64 {
      tunnel: ["Time (Seconds)" ("element") "Time (Minutes)" ("element") "Time (Hours)" ("element")] -> w104
      frame 0 {
      }
      frame 1, Default {
      }
      frame 2 {
      }
    }
    n466 = Build Array(w117, w72, w82, w81, w80, w79, w78, w77, w76, w75, w74, w73, w71) -> (w139:dbl[][])
    n467 = Transpose 2D Array(2D array=w139) -> (transposed array=w138:dbl[][])
    n468 = Concatenate Strings(w69, "-Imax_Imin_Ion_Ioff_vs_time.txt" ("Suffix (Imax,Imin,Ion,Ioff)")) -> (w149:string)
    n469 = Build Array(w104, "Is max (A)" ("VAR2 Name"), "Is min (A)" ("VAR2 Name"), "Id max (A)" ("VAR2 Name"), "Id min (A)" ("VAR2 Name"), "Ig max (A)" ("VAR2 Name"), "Ig min (A)" ("VAR2 Name"), "Is on (A)" ("VAR2 Name"), "Is off (A)" ("VAR2 Name"), "Id on (A)" ("VAR2 Name"), "Id off (A)" ("VAR2 Name"), "Ig on (A)" ("VAR2 Name"), "Ig off (A)" ("VAR2 Name")) -> (w144:string[])
    n470 = Array To Spreadsheet String(array=w138, 3:"%e" ("format string")) -> (spreadsheet string=w142:string)  [unwired: 1 in]
    n471 = Array To Spreadsheet String(array=w144, 3:"" ("format string")) -> (spreadsheet string=w143:string)  [unwired: 1 in]
    n472 = String To Path(string=w149) -> (path=w148:path)
    n473 = Build Array(w143, w142) -> (w141:string[])
    n474 = Write to Text File(file (use dialog)=w148, text=w141, error in=w115) -> (refnum out=w150:refnum<file>, error out=w140:errorcluster)  [unwired: 1 in, 1 out]
    n475 = Close File(refnum=w150, error in=w140) -> (error out=w68:errorcluster)  [unwired: 1 out]
    n476 = Concatenate Strings(w69, "-serial_port_output.txt" ("Suffix (serial port log)")) -> (w119:string)
    n477 = String To Path(string=w119) -> (path=w118:path)
    n478 = Build Array(w104, "Serial port input" ("VAR2 Name"), "Serial port output: ") -> (w108:string[])
    n479 = Array To Spreadsheet String(array=w112, 3:"" ("format string")) -> (spreadsheet string=w105:string)  [unwired: 1 in]
    n480 = Array To Spreadsheet String(array=w108, 3:"" ("format string")) -> (spreadsheet string=w106:string)  [unwired: 1 in]
    n481 = Build Array(w106, w105) -> (w107:string[])
    n482 = Array To Spreadsheet String(array=w111, 3:"" ("format string")) -> (spreadsheet string=w124:string)  [unwired: 1 in]
    n483 = Write to Text File(file (use dialog)=w118, text=w107, error in=w68) -> (refnum out=w120:refnum<file>, error out=w121:errorcluster)  [unwired: 1 in, 1 out]
    n484 = Close File(refnum=w120, error in=w121) -> (error out=w66:errorcluster)  [unwired: 1 out]
    n485 = local write "Serial port data"(w124) -> ()
  }
  "error out" <- w26
  "Timings Indicator" <- w17
  "Is max" <- w11
  "Id max" <- w11
  "Ig max" <- w11
  "Imax vs time" <- w7
  "I vs Vg" <- w7
  "Imin vs time" <- w7
  "I vs Vd" <- w7
  "Serial port data" <- "" ("Serial port data")
  "Is min" <- w10
  "Id min" <- w10
  "Ig min" <- w10
  "Ion vs time" <- w7
  "Ioff vs time" <- w7
  "Is on" <- w9
  "Id on" <- w9
  "Ig on" <- w9
  "Is off" <- w8
  "Id off" <- w8
  "Ig off" <- w8
